vi "DCREG.vi"(10 "Simulazione":bool) -> ()   [LabVIEW 2019]
uses:
  Parametri DCREG letti.ctl
  <vilib>/Utility/file.llb/Read Delimited Spreadsheet (string).vi
  <vilib>/Modbus/master/Create Master Instance (Serial).vi
  Global FINE AVVIO.vi
  <vilib>/Modbus/master/Modbus Master.lvclass
  <vilib>/ptbypt/NI_PtbyPt.lvlib
panel:
  out "# elements in queue":i32
  out "P010 RPM max":dbl
  out "Connesso?":bool=TRUE
  out "Configurazioni dcreg":T1
  out "error out 5":errorcluster
  out "error out 4":errorcluster
  out "error out 3":errorcluster
  out "error out 2":errorcluster
  out "M0018 I CAMPO [A]":dbl
  out "M006 V ARMATURA [V]":dbl
  out "M004 I ARMATURA [A]":dbl
  out "P011 Vdc arm NOM":dbl
  in  "config":bool
  in  "Config DCreg":T1
  in  "IECC":dbl
  in  "SET IECC":bool
  in  "set rampa":bool
  in  "Rampa s":dbl
  in  "set Iarm":bool
  in  "Inom arm":dbl
  in  "set varm":bool
  in  "Vdc arm":dbl
  in  "disconnetti":bool
  in  "connetti":bool
  out "Iecc":dbl
  out "Iecc":dbl
  out "Imax mot":dbl
  out "Vdcreg":dbl
  in  "Leggi tutto?":bool
  out "P[KW]":dbl
  out "I[A]":dbl
  out "V[V]":dbl
  out "error out":errorcluster
  out "DCREG":T2
  in  "starting address":u16
  in  "holding register values":u16[](array[numeric])
  out "t":errorcluster
  out "N°reg_ValReg":i32[][](array[numeric])
  in  "mostra num registro":bool
  in  "SETUP PORTA SERIALE":T3={"Porta COM"="COM8", "Baud Rate"=38400, "Parity"=0, "Flow Control"=0, "Timeout"=10000, "Mode"=enum."RTU", "Slave Address"=2} {"Flow Control" items=["None", "XON/XOFF", "RTS/CTS", "XON/XOFF & RTS/CTS", "DTR/DSR", "XON/XOFF & DTR/DSR"]; "Parity" items=["None", "Odd", "Even", "Mark", "Space"]}
  out "STATO":string
  out "Numeric":i32
  in  "stop":bool
  in  "write register":bool
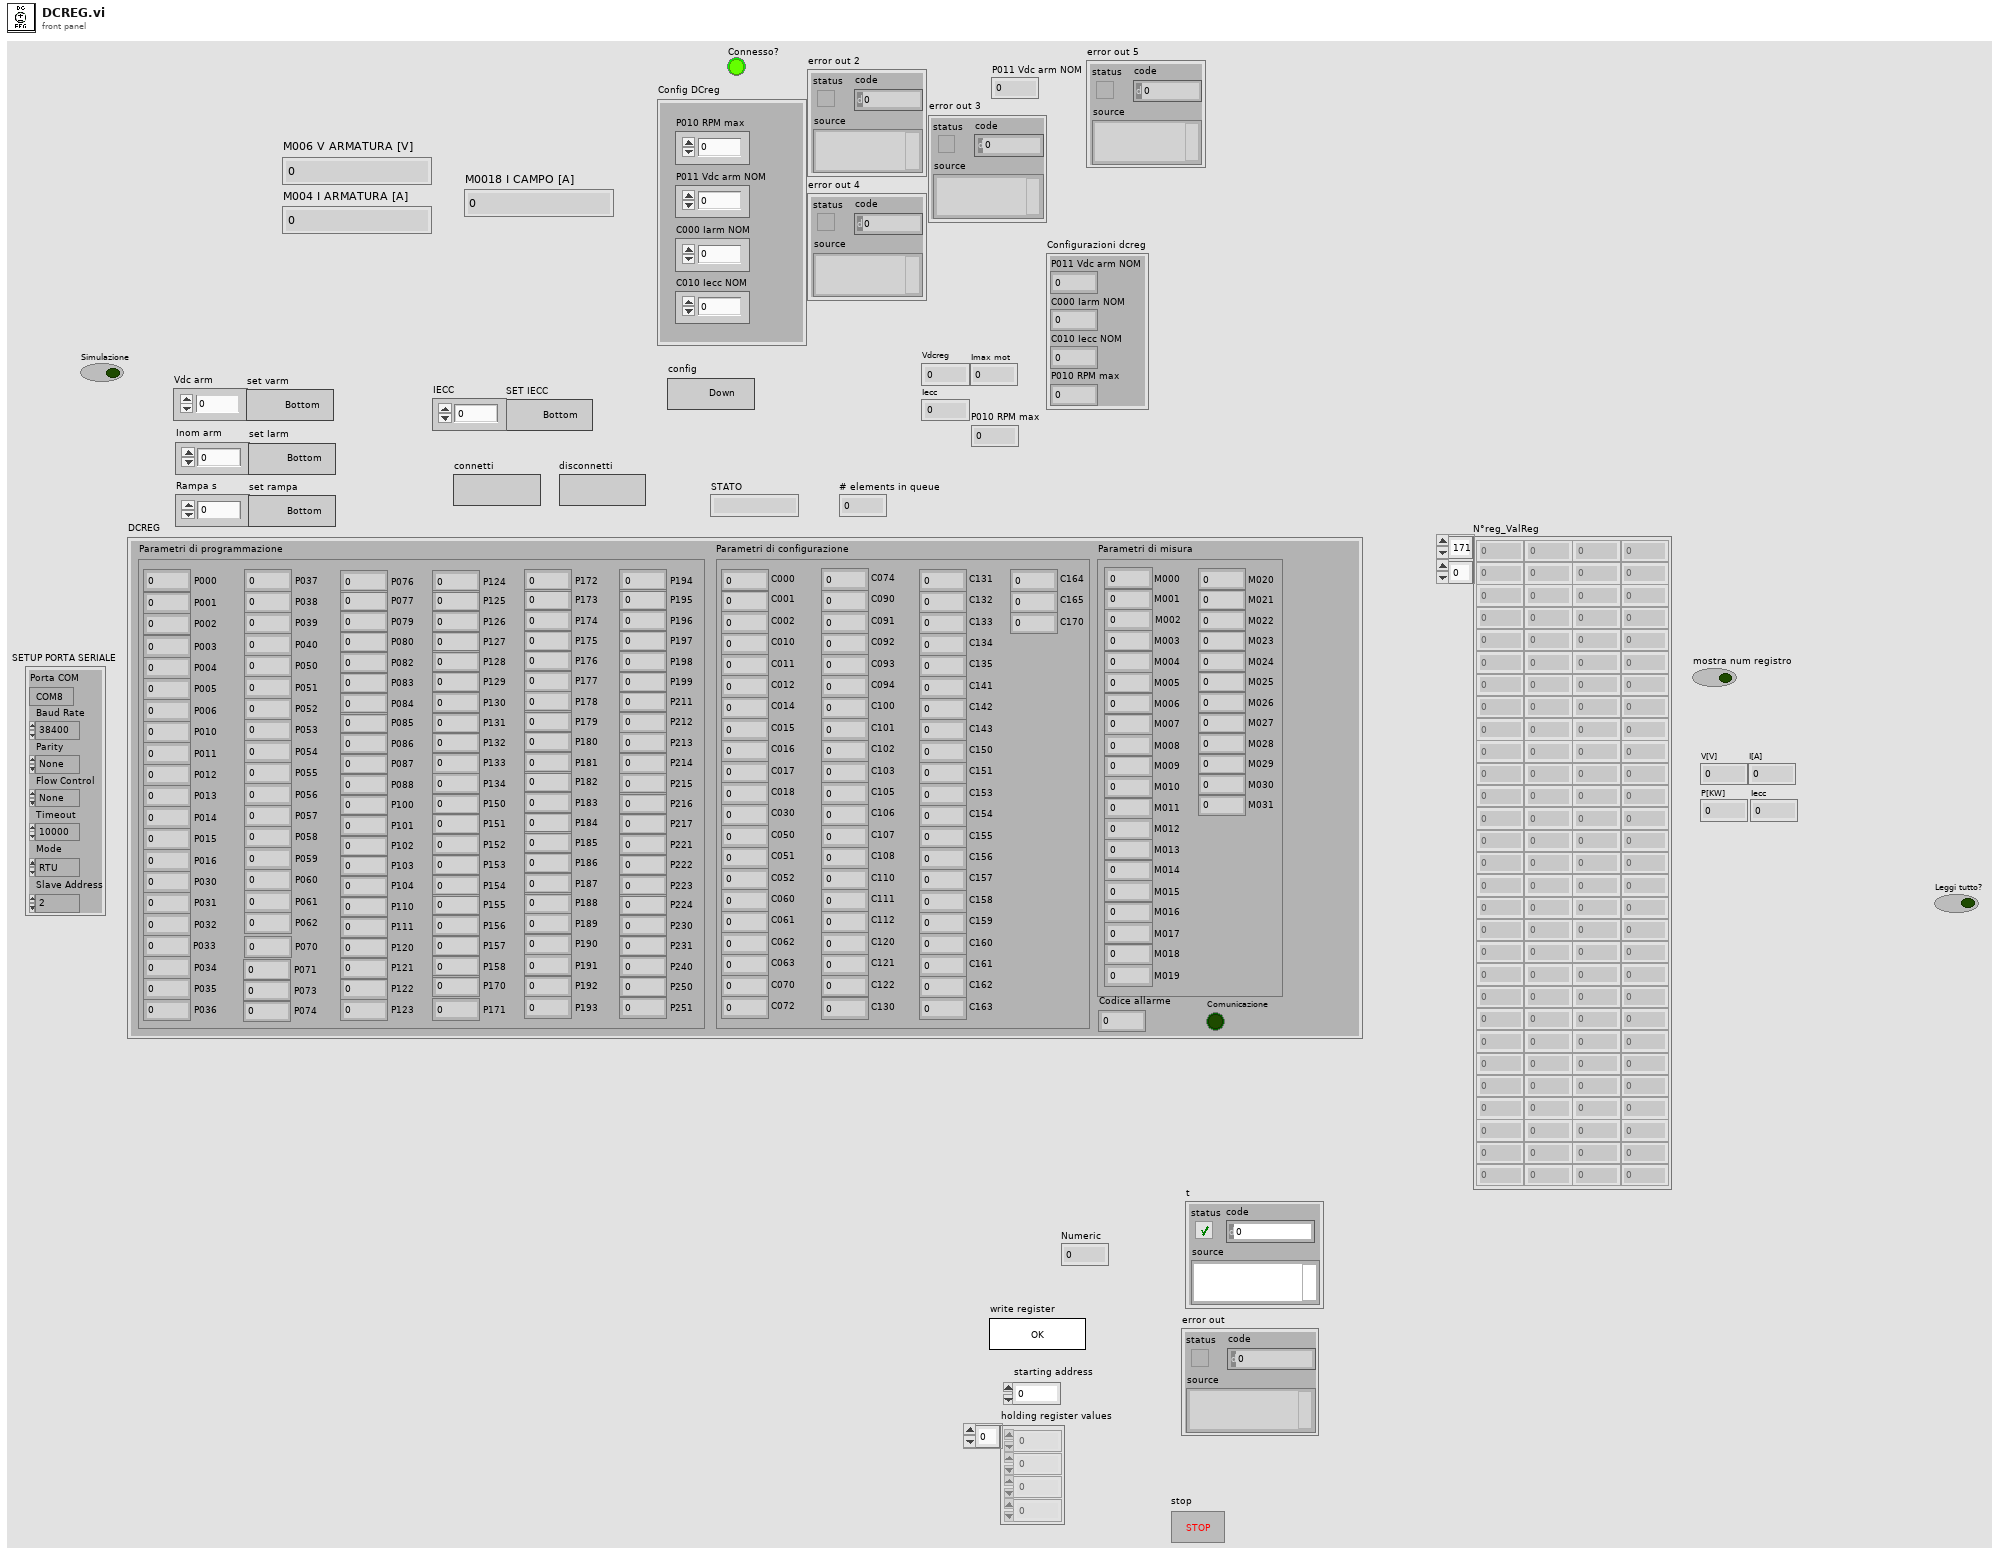
[diagram p1: front panel]
types:
  T1 = cluster{"P011 Vdc arm NOM":dbl, "C000 Iarm NOM":dbl, "C010 Iecc NOM":dbl, "P010 RPM max":dbl}
  T2 = typedef "Parametri DCREG letti.ctl" = cluster{"Parametri di misura":cluster{"M000":dbl, "M001":dbl, "M002":dbl, "M003":dbl, "M004":dbl, "M005":dbl, "M006":dbl, "M007":dbl, "M008":dbl, "M009":dbl, "M010":dbl, "M011":dbl, "M012":dbl, "M013":dbl, "M014":dbl, "M015":dbl, "M016":dbl, "M017":dbl, "M018":dbl, "M019":dbl, "M020":dbl, "M021":dbl, "M022":dbl, "M023":dbl, "M024":dbl, "M025":dbl, "M026":dbl, "M027":dbl, "M028":dbl, "M029":dbl, "M030":dbl, "M031":dbl}, "Parametri di programmazione":cluster{"P000":dbl, "P001":dbl, "P002":dbl, "P003":dbl, "P004":dbl, "P005":dbl, "P006":dbl, "P010":dbl, "P011":dbl, "P012":dbl, "P013":dbl, "P014":dbl, "P015":dbl, "P016":dbl, "P030":dbl, "P031":dbl, "P032":dbl, "P033":dbl, "P034":dbl, "P035":dbl, "P036":dbl, "P037":dbl, "P038":dbl, "P039":dbl, "P040":dbl, "P050":dbl, "P051":dbl, "P052":dbl, "P053":dbl, "P054":dbl, "P055":dbl, "P056":dbl, "P057":dbl, "P058":dbl, "P059":dbl, "P060":dbl, "P061":dbl, "P062":dbl, "P070":dbl, "P071":dbl, "P073":dbl, "P074":dbl, "P076":dbl, "P077":dbl, "P079":dbl, "P080":dbl, "P082":dbl, "P083":dbl, "P084":dbl, "P085":dbl, "P086":dbl, "P087":dbl, "P088":dbl, "P100":dbl, "P101":dbl, "P102":dbl, "P103":dbl, "P104":dbl, "P110":dbl, "P111":dbl, "P120":dbl, "P121":dbl, "P122":dbl, "P123":dbl, "P124":dbl, "P125":dbl, "P126":dbl, "P127":dbl, "P128":dbl, "P129":dbl, "P130":dbl, "P131":dbl, "P132":dbl, "P133":dbl, "P134":dbl, "P150":dbl, "P151":dbl, "P152":dbl, "P153":dbl, "P154":dbl, "P155":dbl, "P156":dbl, "P157":dbl, "P158":dbl, "P170":dbl, "P171":dbl, "P172":dbl, "P173":dbl, "P174":dbl, "P175":dbl, "P176":dbl, "P177":dbl, "P178":dbl, "P179":dbl, "P180":dbl, "P181":dbl, "P182":dbl, "P183":dbl, "P184":dbl, "P185":dbl, "P186":dbl, "P187":dbl, "P188":dbl, "P189":dbl, "P190":dbl, "P191":dbl, "P192":dbl, "P193":dbl, "P194":dbl, "P195":dbl, "P196":dbl, "P197":dbl, "P198":dbl, "P199":dbl, "P211":dbl, "P212":dbl, "P213":dbl, "P214":dbl, "P215":dbl, "P216":dbl, "P217":dbl, "P221":dbl, "P222":dbl, "P223":dbl, "P224":dbl, "P230":dbl, "P231":dbl, "P240":dbl, "P250":dbl, "P251":dbl}, "Parametri di configurazione":cluster{"C000":dbl, "C001":dbl, "C002":dbl, "C010":dbl, "C011":dbl, "C012":dbl, "C014":dbl, "C015":dbl, "C016":dbl, "C017":dbl, "C018":dbl, "C030":dbl, "C050":dbl, "C051":dbl, "C052":dbl, "C060":dbl, "C061":dbl, "C062":dbl, "C063":dbl, "C070":dbl, "C072":dbl, "C074":dbl, "C090":dbl, "C091":dbl, "C092":dbl, "C093":dbl, "C094":dbl, "C100":dbl, "C101":dbl, "C102":dbl, "C103":dbl, "C105":dbl, "C106":dbl, "C107":dbl, "C108":dbl, "C110":dbl, "C111":dbl, "C112":dbl, "C120":dbl, "C121":dbl, "C122":dbl, "C130":dbl, "C131":dbl, "C132":dbl, "C133":dbl, "C134":dbl, "C135":dbl, "C141":dbl, "C142":dbl, "C143":dbl, "C150":dbl, "C151":dbl, "C153":dbl, "C154":dbl, "C155":dbl, "C156":dbl, "C157":dbl, "C158":dbl, "C159":dbl, "C160":dbl, "C161":dbl, "C162":dbl, "C163":dbl, "C164":dbl, "C165":dbl, "C170":dbl}, "Codice allarme":dbl, "Comunicazione":bool}
  T3 = cluster{"Porta COM":string, "Baud Rate":u32, "Parity":u16, "Flow Control":u16, "Timeout":u32, "Mode":enum16{"RTU", "ASCII"}, "Slave Address":u8}
  T4 = cluster{"Array of elements":cluster{"String":string, "variant":variant}[], "Single element":cluster{"String":string, "variant":variant}, "enque at\nopposite end (F)":bool, "no replications (F)":bool}
  T5 = cluster{"P000":dbl, "P001":dbl, "P002":dbl, "P003":dbl, "P004":dbl, "P005":dbl, "P006":dbl, "P010":dbl, "P011":dbl, "P012":dbl, "P013":dbl, "P014":dbl, "P015":dbl, "P016":dbl, "P030":dbl, "P031":dbl, "P032":dbl, "P033":dbl, "P034":dbl, "P035":dbl, "P036":dbl, "P037":dbl, "P038":dbl, "P039":dbl, "P040":dbl, "P050":dbl, "P051":dbl, "P052":dbl, "P053":dbl, "P054":dbl, "P055":dbl, "P056":dbl, "P057":dbl, "P058":dbl, "P059":dbl, "P060":dbl, "P061":dbl, "P062":dbl, "P070":dbl, "P071":dbl, "P073":dbl, "P074":dbl, "P076":dbl, "P077":dbl, "P079":dbl, "P080":dbl, "P082":dbl, "P083":dbl, "P084":dbl, "P085":dbl, "P086":dbl, "P087":dbl, "P088":dbl, "P100":dbl, "P101":dbl, "P102":dbl, "P103":dbl, "P104":dbl, "P110":dbl, "P111":dbl, "P120":dbl, "P121":dbl, "P122":dbl, "P123":dbl, "P124":dbl, "P125":dbl, "P126":dbl, "P127":dbl, "P128":dbl, "P129":dbl, "P130":dbl, "P131":dbl, "P132":dbl, "P133":dbl, "P134":dbl, "P150":dbl, "P151":dbl, "P152":dbl, "P153":dbl, "P154":dbl, "P155":dbl, "P156":dbl, "P157":dbl, "P158":dbl, "P170":dbl, "P171":dbl, "P172":dbl, "P173":dbl, "P174":dbl, "P175":dbl, "P176":dbl, "P177":dbl, "P178":dbl, "P179":dbl, "P180":dbl, "P181":dbl, "P182":dbl, "P183":dbl, "P184":dbl, "P185":dbl, "P186":dbl, "P187":dbl, "P188":dbl, "P189":dbl, "P190":dbl, "P191":dbl, "P192":dbl, "P193":dbl, "P194":dbl, "P195":dbl, "P196":dbl, "P197":dbl, "P198":dbl, "P199":dbl, "P211":dbl, "P212":dbl, "P213":dbl, "P214":dbl, "P215":dbl, "P216":dbl, "P217":dbl, "P221":dbl, "P222":dbl, "P223":dbl, "P224":dbl, "P230":dbl, "P231":dbl, "P240":dbl, "P250":dbl, "P251":dbl}
  T6 = cluster{"C000":dbl, "C001":dbl, "C002":dbl, "C010":dbl, "C011":dbl, "C012":dbl, "C014":dbl, "C015":dbl, "C016":dbl, "C017":dbl, "C018":dbl, "C030":dbl, "C050":dbl, "C051":dbl, "C052":dbl, "C060":dbl, "C061":dbl, "C062":dbl, "C063":dbl, "C070":dbl, "C072":dbl, "C074":dbl, "C090":dbl, "C091":dbl, "C092":dbl, "C093":dbl, "C094":dbl, "C100":dbl, "C101":dbl, "C102":dbl, "C103":dbl, "C105":dbl, "C106":dbl, "C107":dbl, "C108":dbl, "C110":dbl, "C111":dbl, "C112":dbl, "C120":dbl, "C121":dbl, "C122":dbl, "C130":dbl, "C131":dbl, "C132":dbl, "C133":dbl, "C134":dbl, "C135":dbl, "C141":dbl, "C142":dbl, "C143":dbl, "C150":dbl, "C151":dbl, "C153":dbl, "C154":dbl, "C155":dbl, "C156":dbl, "C157":dbl, "C158":dbl, "C159":dbl, "C160":dbl, "C161":dbl, "C162":dbl, "C163":dbl, "C164":dbl, "C165":dbl, "C170":dbl}
  T7 = cluster{"M000":dbl, "M001":dbl, "M002":dbl, "M003":dbl, "M004":dbl, "M005":dbl, "M006":dbl, "M007":dbl, "M008":dbl, "M009":dbl, "M010":dbl, "M011":dbl, "M012":dbl, "M013":dbl, "M014":dbl, "M015":dbl, "M016":dbl, "M017":dbl, "M018":dbl, "M019":dbl, "M020":dbl, "M021":dbl, "M022":dbl, "M023":dbl, "M024":dbl, "M025":dbl, "M026":dbl, "M027":dbl, "M028":dbl, "M029":dbl, "M030":dbl, "M031":dbl}
  T8 = cluster{"C011":dbl, "C012":dbl, "C016":dbl, "Conferma":bool}
  T9 = cluster{"[0]":i32, "[1]":i32, "[2]":i32, "[3]":i32, "[4]":i32, "[5]":i32, "[6]":i32, "[7]":i32, "[8]":i32, "[9]":i32, "[10]":i32, "[11]":i32, "[12]":i32, "[13]":i32, "[14]":i32, "[15]":i32, "[16]":i32, "[17]":i32, "[18]":i32, "[19]":i32, "[20]":i32, "[21]":i32, "[22]":i32, "[23]":i32, "[24]":i32, "[25]":i32, "[26]":i32, "[27]":i32, "[28]":i32, "[29]":i32, "[30]":i32, "[31]":i32}
  T10 = cluster{"[0]":i32, "[1]":i32, "[2]":i32, "[3]":i32, "[4]":i32, "[5]":i32, "[6]":i32, "[7]":i32, "[8]":i32, "[9]":i32, "[10]":i32, "[11]":i32, "[12]":i32, "[13]":i32, "[14]":i32, "[15]":i32, "[16]":i32, "[17]":i32, "[18]":i32, "[19]":i32, "[20]":i32, "[21]":i32, "[22]":i32, "[23]":i32, "[24]":i32, "[25]":i32, "[26]":i32, "[27]":i32, "[28]":i32, "[29]":i32, "[30]":i32, "[31]":i32, "[32]":i32, "[33]":i32, "[34]":i32, "[35]":i32, "[36]":i32, "[37]":i32, "[38]":i32, "[39]":i32, "[40]":i32, "[41]":i32, "[42]":i32, "[43]":i32, "[44]":i32, "[45]":i32, "[46]":i32, "[47]":i32, "[48]":i32, "[49]":i32, "[50]":i32, "[51]":i32, "[52]":i32, "[53]":i32, "[54]":i32, "[55]":i32, "[56]":i32, "[57]":i32, "[58]":i32, "[59]":i32, "[60]":i32, "[61]":i32, "[62]":i32, "[63]":i32, "[64]":i32, "[65]":i32, "[66]":i32, "[67]":i32, "[68]":i32, "[69]":i32, "[70]":i32, "[71]":i32, "[72]":i32, "[73]":i32, "[74]":i32, "[75]":i32, "[76]":i32, "[77]":i32, "[78]":i32, "[79]":i32, "[80]":i32, "[81]":i32, "[82]":i32, "[83]":i32, "[84]":i32, "[85]":i32, "[86]":i32, "[87]":i32, "[88]":i32, "[89]":i32, "[90]":i32, "[91]":i32, "[92]":i32, "[93]":i32, "[94]":i32, "[95]":i32, "[96]":i32, "[97]":i32, "[98]":i32, "[99]":i32, "[100]":i32, "[101]":i32, "[102]":i32, "[103]":i32, "[104]":i32, "[105]":i32, "[106]":i32, "[107]":i32, "[108]":i32, "[109]":i32, "[110]":i32, "[111]":i32, "[112]":i32, "[113]":i32, "[114]":i32, "[115]":i32, "[116]":i32, "[117]":i32, "[118]":i32, "[119]":i32, "[120]":i32, "[121]":i32, "[122]":i32, "[123]":i32, "[124]":i32, "[125]":i32, "[126]":i32, "[127]":i32, "[128]":i32, "[129]":i32}
  T11 = cluster{"[0]":i32, "[1]":i32, "[2]":i32, "[3]":i32, "[4]":i32, "[5]":i32, "[6]":i32, "[7]":i32, "[8]":i32, "[9]":i32, "[10]":i32, "[11]":i32, "[12]":i32, "[13]":i32, "[14]":i32, "[15]":i32, "[16]":i32, "[17]":i32, "[18]":i32, "[19]":i32, "[20]":i32, "[21]":i32, "[22]":i32, "[23]":i32, "[24]":i32, "[25]":i32, "[26]":i32, "[27]":i32, "[28]":i32, "[29]":i32, "[30]":i32, "[31]":i32, "[32]":i32, "[33]":i32, "[34]":i32, "[35]":i32, "[36]":i32, "[37]":i32, "[38]":i32, "[39]":i32, "[40]":i32, "[41]":i32, "[42]":i32, "[43]":i32, "[44]":i32, "[45]":i32, "[46]":i32, "[47]":i32, "[48]":i32, "[49]":i32, "[50]":i32, "[51]":i32, "[52]":i32, "[53]":i32, "[54]":i32, "[55]":i32, "[56]":i32, "[57]":i32, "[58]":i32, "[59]":i32, "[60]":i32, "[61]":i32, "[62]":i32, "[63]":i32, "[64]":i32, "[65]":i32}
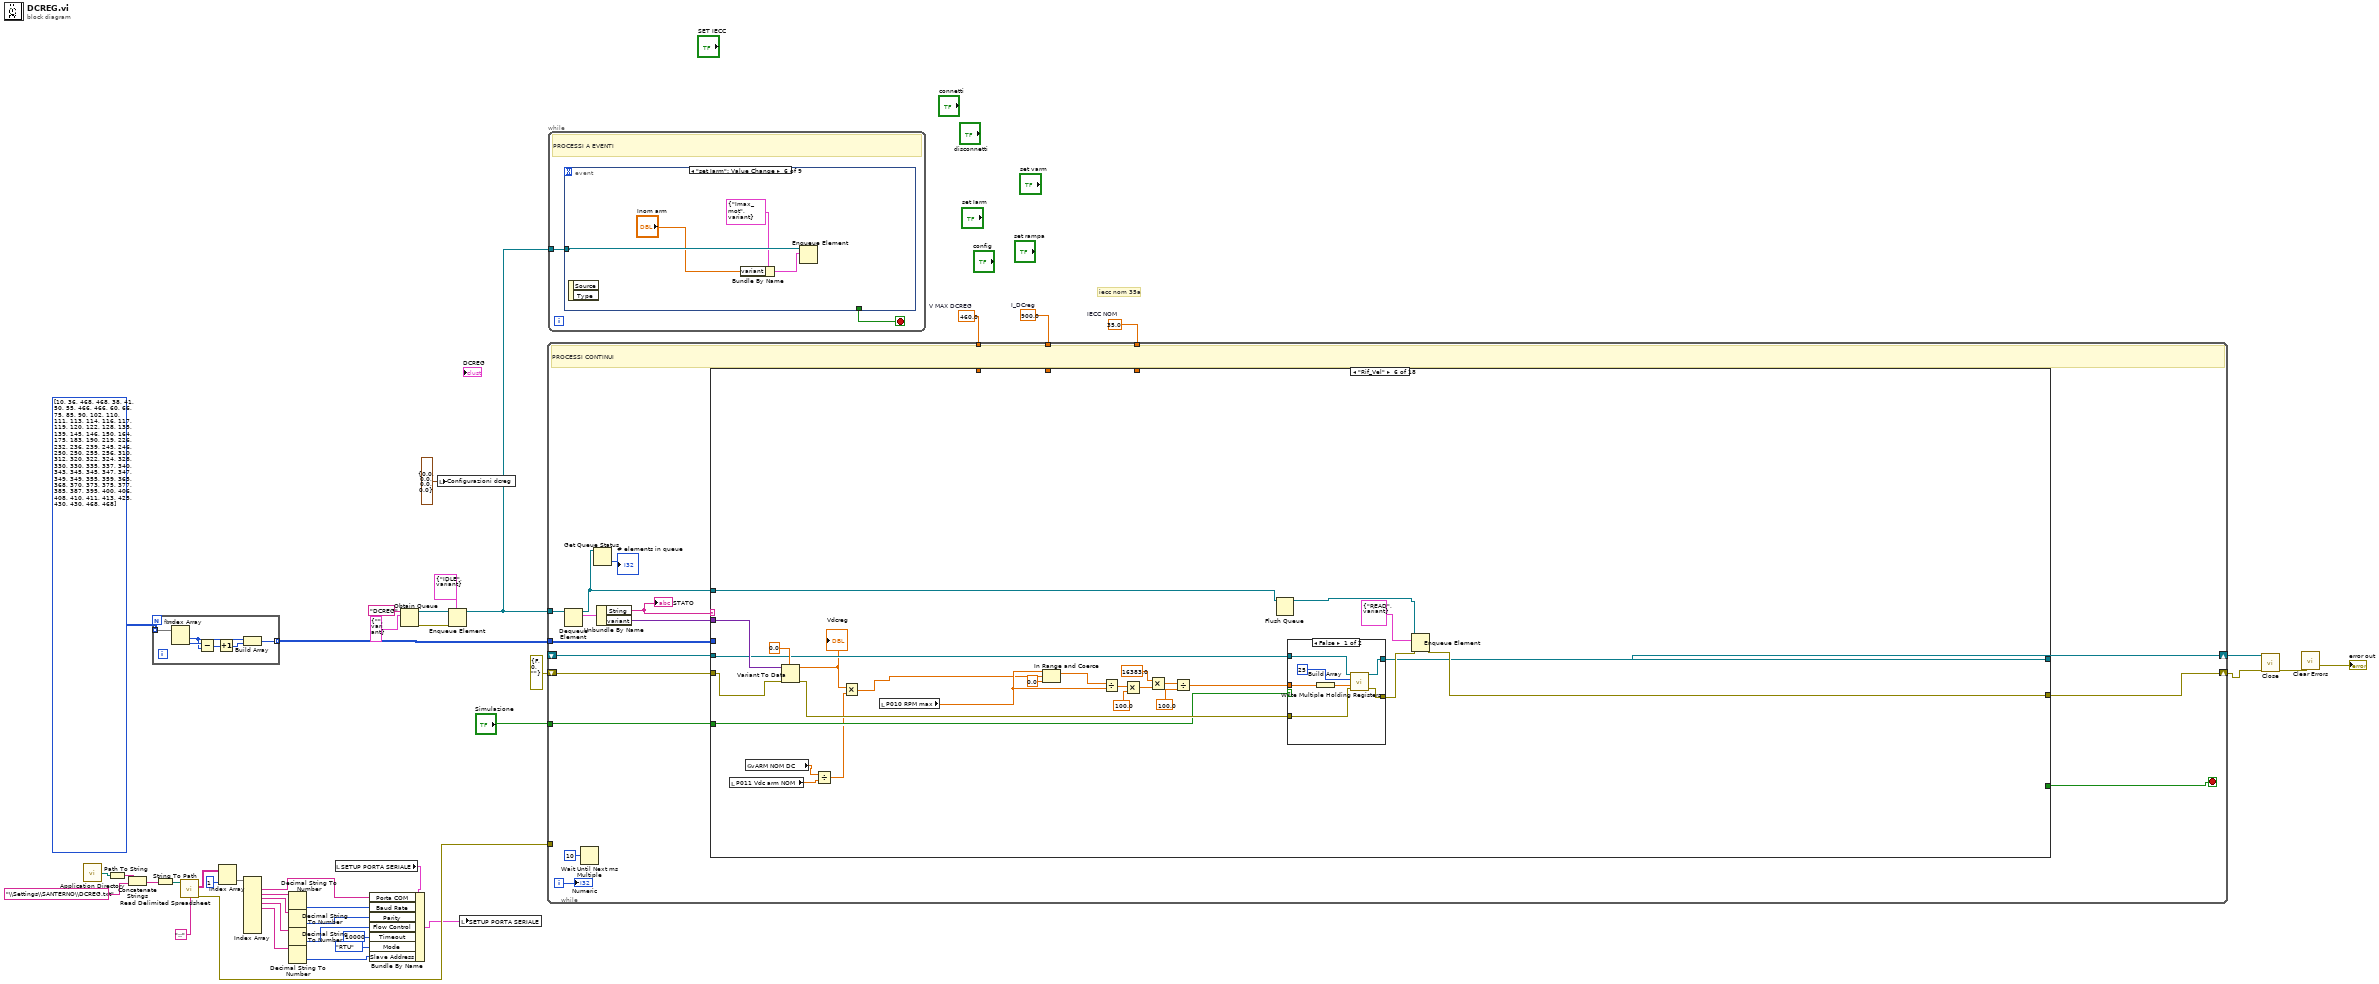
[diagram p0: block diagram]
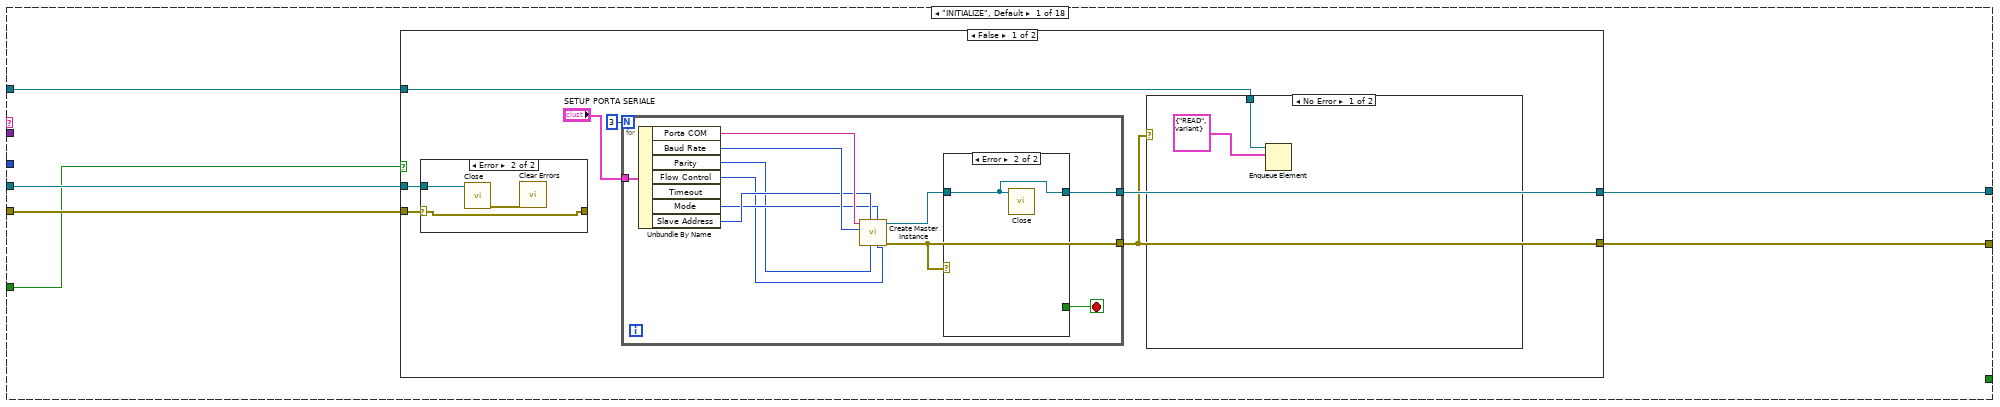
[diagram p2: hidden frame]
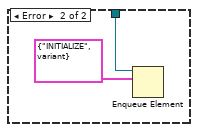
[diagram p3: hidden frame]
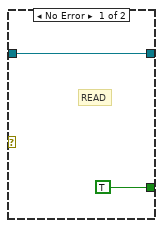
[diagram p5: hidden frame]
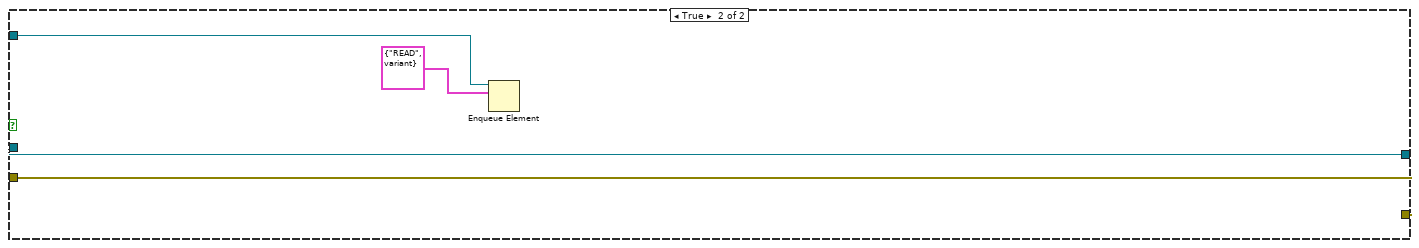
[diagram p6: hidden frame]
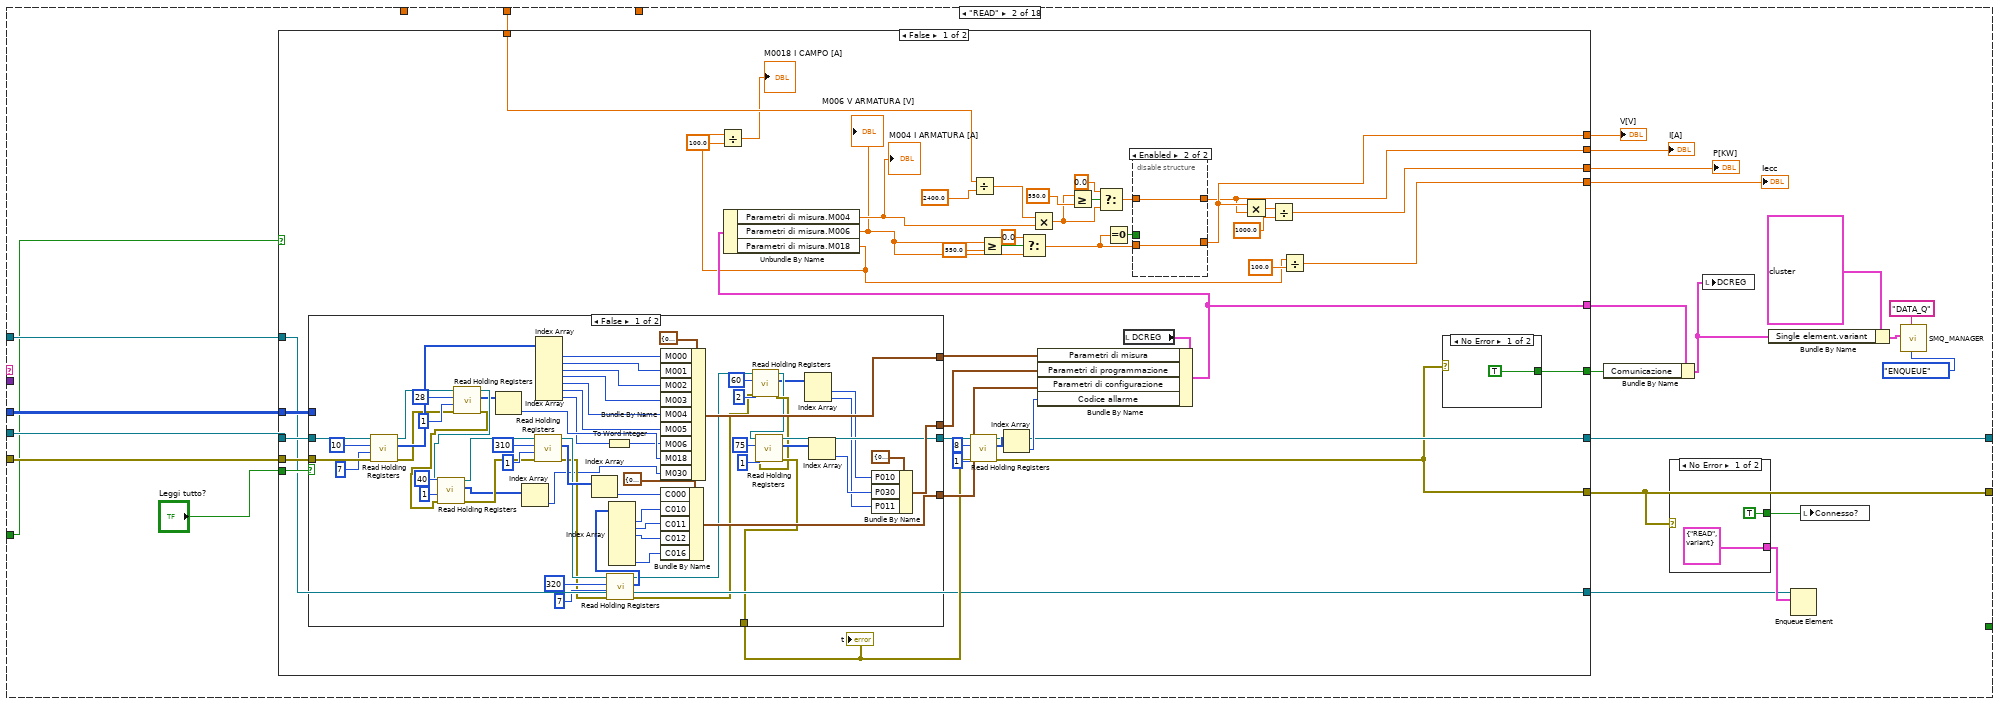
[diagram p7: hidden frame]
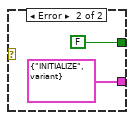
[diagram p8: hidden frame]
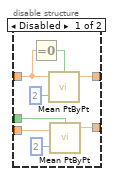
[diagram p10: hidden frame]
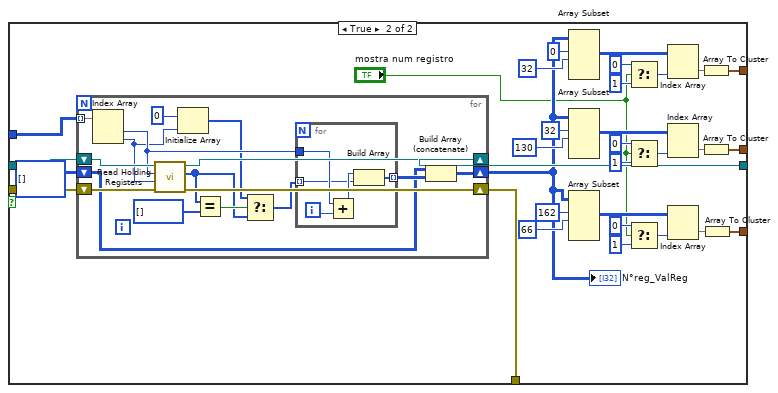
[diagram p11: hidden frame]
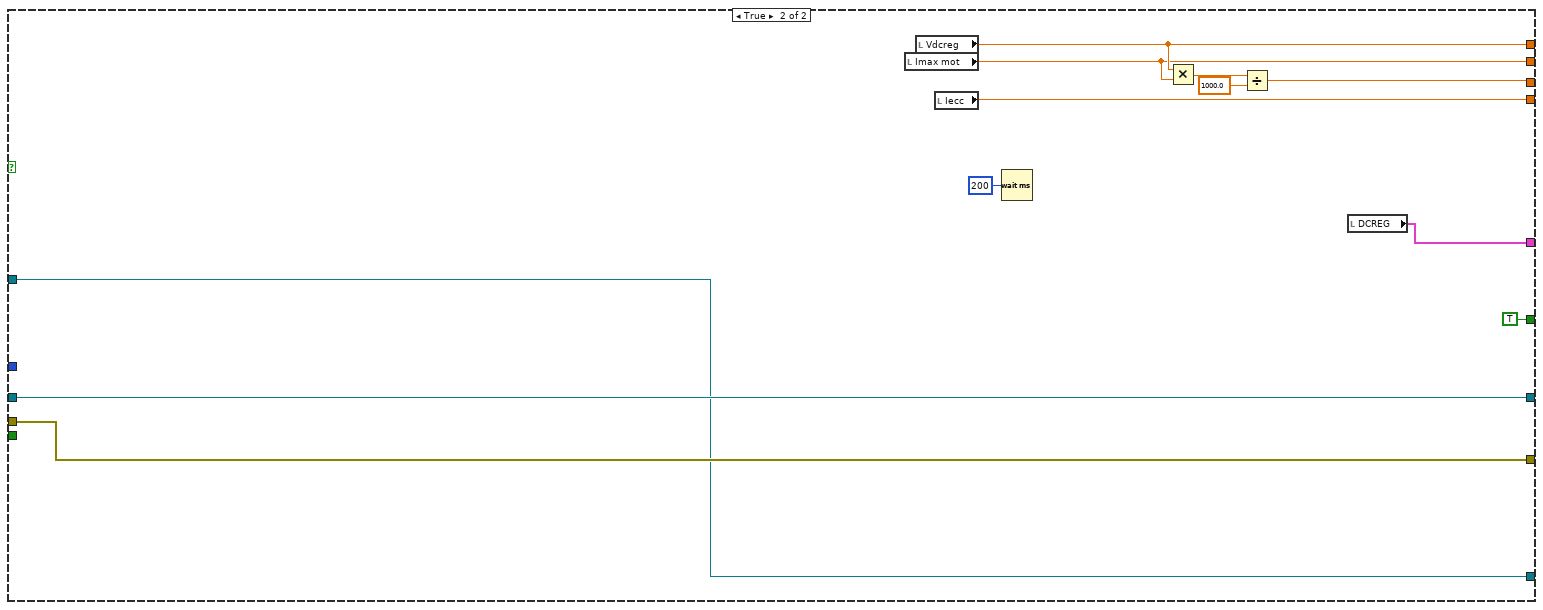
[diagram p12: hidden frame]
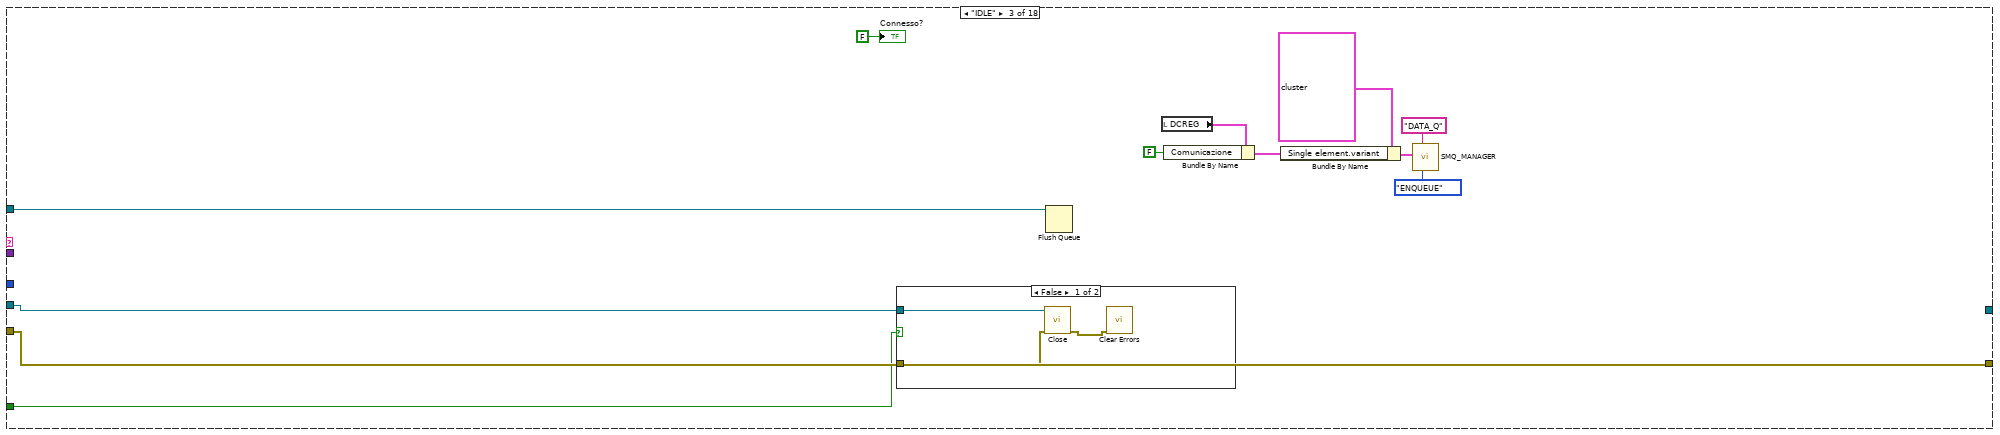
[diagram p13: hidden frame]
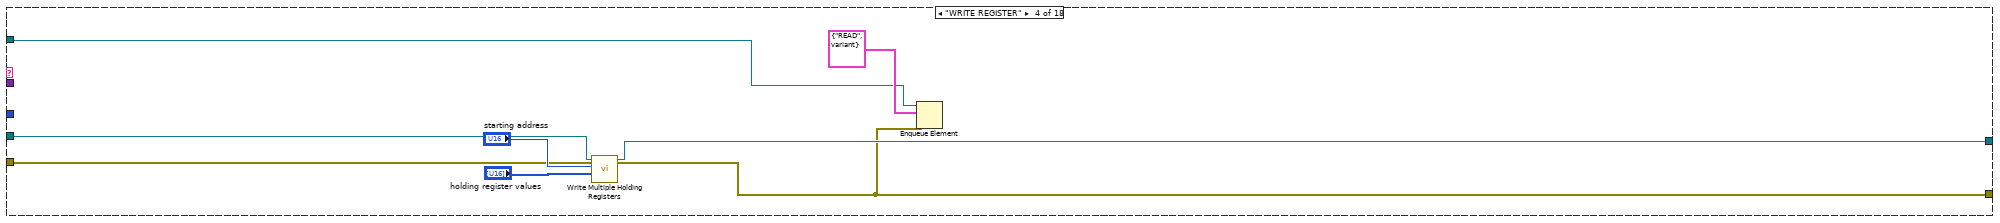
[diagram p15: hidden frame]
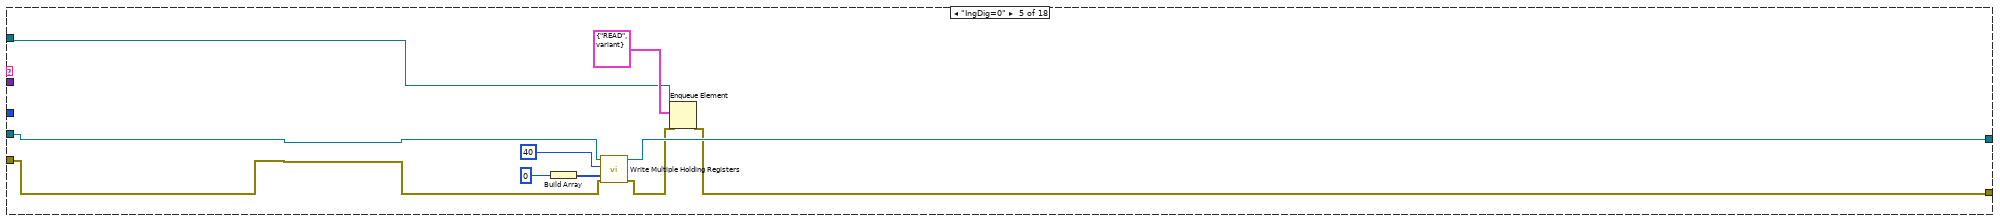
[diagram p16: hidden frame]
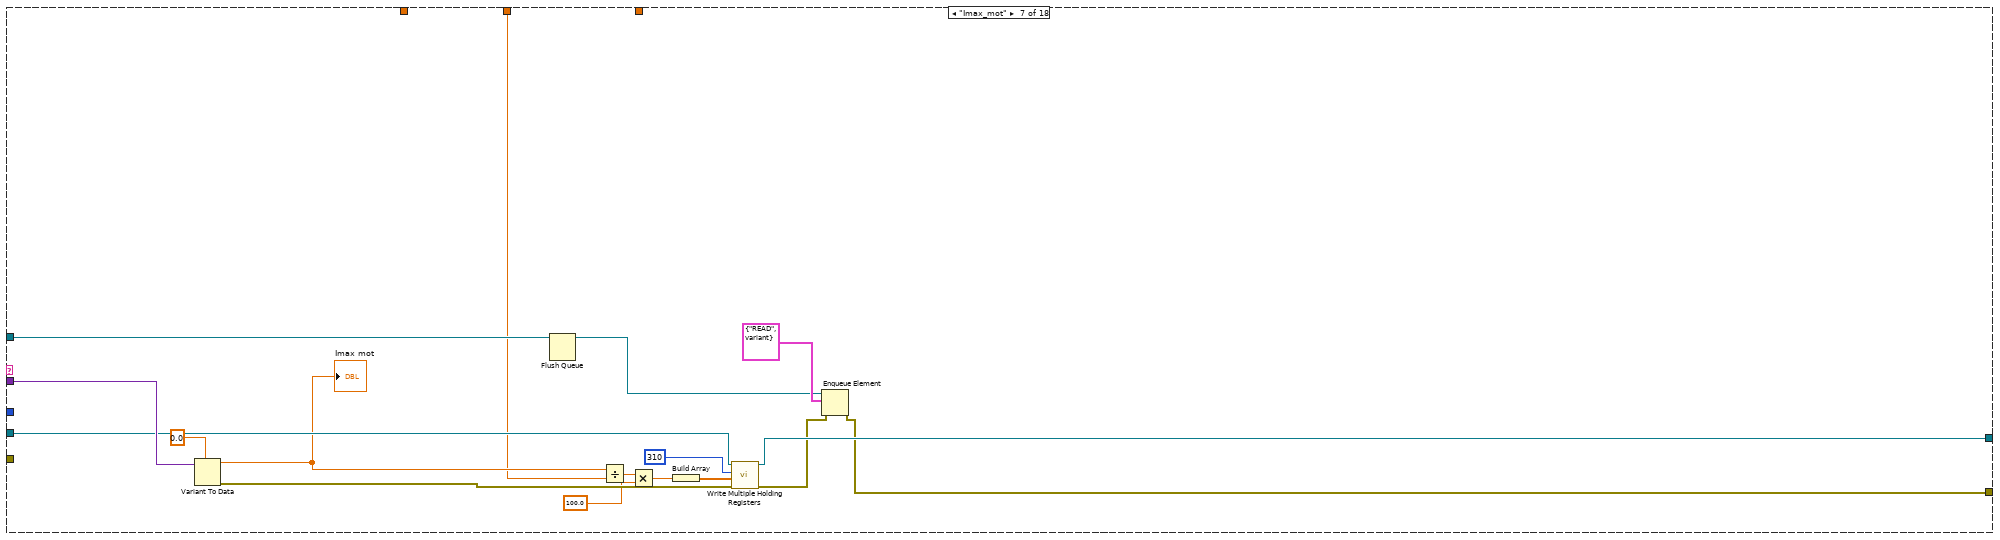
[diagram p18: hidden frame]
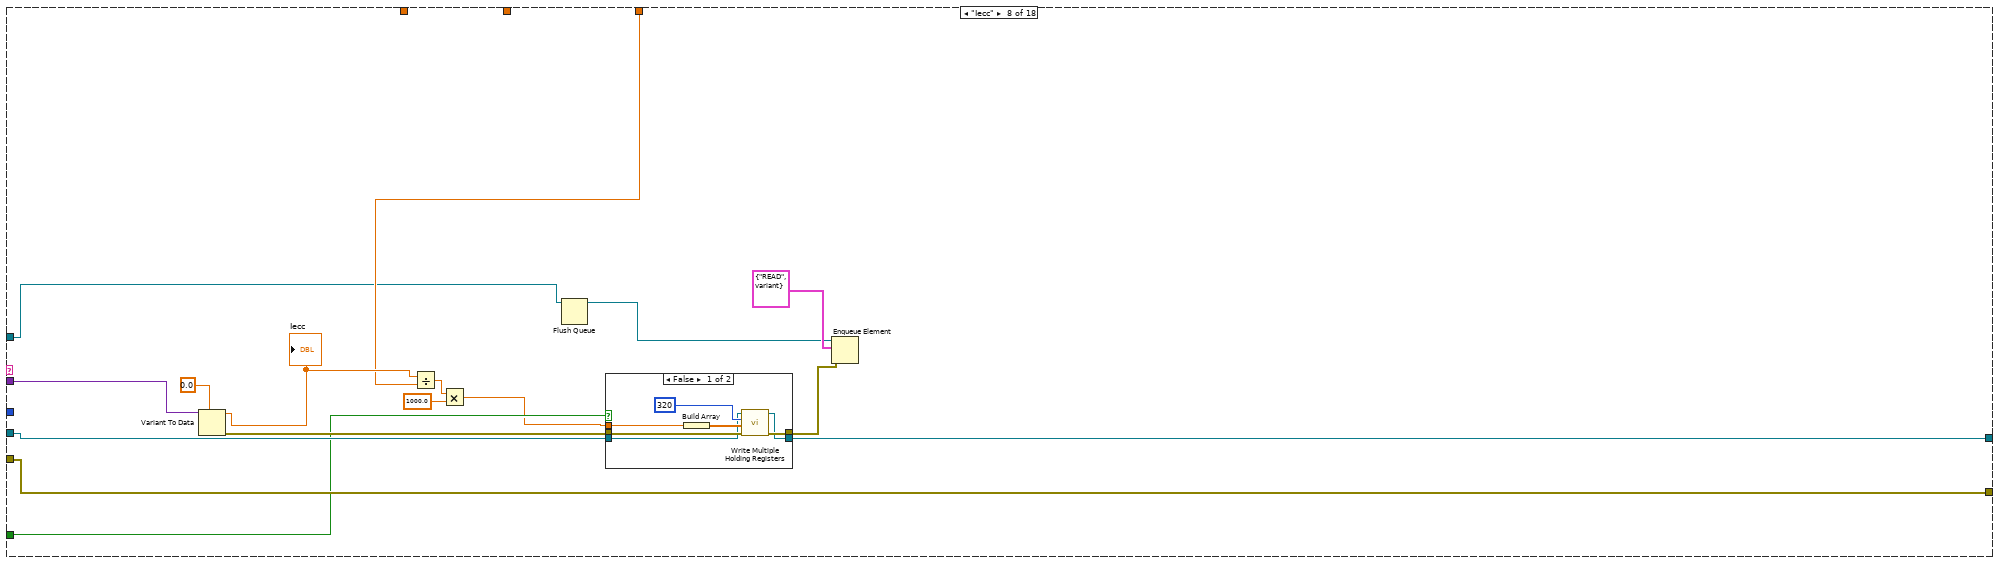
[diagram p19: hidden frame]
diagram:
  w25 = 35.0  # IECC NOM
  w29 = 900.0  # I_DCreg
  w30 = 460.0  # V MAX DCREG
  # "iecc nom 35a"
  n1 = call <vilib>:"Application Directory.vi"() -> ("Application Directory"=w12:path)
  n2 = Path To String(path=w12) -> (string=w13:string)
  n3 = Concatenate Strings(w13, "\\Settings\\SANTERNO\\DCREG.txt" ("string")) -> (w15:string)
  n4 = for {
    tunnel: i32[][] [[10, 36], [468, 468], [38, 41], [50, 55], [466, 466], [60, 66], [75, 85], [90, 102], [110, 111], [113, 114], [116, 117], [119, 120], [122, 128], [135, 139], [145, 146], [150, 164], [175, 183], [190, 219], [226, 232], [236, 239], [245, 246], [250, 250], [255, 256], [310, 312], [320, 322], [324, 328], [330, 330], [335, 337], [340, 343], [345, 345], [347, 347], [349, 349], [355, 359], [365, 368], [370, 373], [375, 377], [385, 387], [395, 400], [406, 408], [410, 411], [413, 425], [430, 430], [468, 468]] -> [w47] mode=indexing
    tunnel: [w42] -> w39 mode=indexing
    n5 = Index Array(array=w47) -> (element #1=w43:i32, element #2=w46:i32)  [unwired: 2 in]
    n6 = Subtract(x=w46, y=w43) -> (x-y=w45:i32)
    n7 = Increment(x=w45) -> (x+1=w44:i32)
    n8 = Build Array(w43, w44) -> (w42:i32[])
  }
  n9 = String To Path(string=w15) -> (path=w16:path)
  n10 = call-poly <vilib>:"Read Delimited Spreadsheet.vi"("file path (dialog if empty)"=w16, "delimiter (\\t)"="::" ("delimiter (\\t)")) -> ("all rows"=w17:string[][], "error out"=w3:errorcluster)  [unwired: 8 in, 4 out]
  n11 = Index Array(array=w17, index (col)=1 ("disabled index (col)")) -> (element=w19:string[])  [unwired: 1 in]
  n12 = Index Array(array=w19) -> (element #1=w10:string, element #2=w20:string, element #3=w21:string, element #4=w22:string, element #5=w23:string)  [unwired: 10 in, 5 out]
  n13 = Decimal String To Number(string=w20) -> (number=w9:i32)  [unwired: 2 in, 1 out]
  n14 = Decimal String To Number(string=w21) -> (number=w8:i32)  [unwired: 2 in, 1 out]
  n15 = Decimal String To Number(string=w22) -> (number=w7:i32)  [unwired: 2 in, 1 out]
  n16 = Decimal String To Number(string=w23) -> (number=w5:i32)  [unwired: 2 in, 1 out]
  n17 = local read "SETUP PORTA SERIALE"() -> (w1:T3)
  n18 = Bundle By Name(cluster=w1, "Porta COM"=w10, "Baud Rate"=w9, "Parity"=w8, "Flow Control"=w7, "Timeout"=u32 10000, "Mode"=enum16{"RTU", "ASCII"}."RTU", "Slave Address"=w5) -> (w2:T3)
  n19 = Obtain Queue(name (unnamed)="DCREG", element data type=cluster{"String":string, "variant":variant} {"String"="", "variant"=variant} ("element")) -> (queue out=w31:refnum<queue>, error out=w33:errorcluster)  [unwired: 3 in, 1 out]
  n20 = local write "Configurazioni dcreg"(T1 {"P011 Vdc arm NOM"=0.0, "C000 Iarm NOM"=0.0, "C010 Iecc NOM"=0.0, "P010 RPM max"=0.0} ("Configurazioni dcreg")) -> ()
  n21 = Enqueue Element(queue=w31, element=cluster{"String":string, "variant":variant} {"String"="IDLE", "variant"=variant}, error in (no error)=w33) -> (queue out=w41:refnum<queue>)  [unwired: 1 in, 2 out]
  n22 = local write "SETUP PORTA SERIALE"(w2) -> ()
  n23 = while {
    shift-right: [w57] -> w37
    shift-left: errorcluster {"status"=FALSE, "code"=0, "source"=""} ("error out") -> [w65]
    tunnel: w41 -> [w55]
    shift-right: [w63] -> w38
    shift-left: _ -> [w62]
    tunnel: w39 -> [w61]
    tunnel: w30 -> [w59]
    tunnel: w29 -> [w58]
    tunnel: "Simulazione" -> [w51]
    tunnel: w25 -> [w50]
    tunnel: w3 -> [_]
    i -> [w64]
    stop <- w56 stop-if-true
    # "PROCESSI CONTINUI"
    n24 = Dequeue Element(queue=w55) -> (queue out=w49:refnum<queue>, element=w54:cluster{"String":string, "variant":variant})  [unwired: 2 in, 2 out]
    n25 = Wait Until Next ms Multiple(millisecond multiple=u32 10 ("milliseconds to wait")) -> ()  [unwired: 1 out]
    n26 = Get Queue Status(queue=w49) -> (# elements in queue=→"# elements in queue":i32)  [unwired: 2 in, 7 out]
    n27 = Unbundle By Name(w54) -> ("String"=w53:string, "variant"=w52:variant)
    "STATO" <- w53
    n28 = case shown="\"Rif_Vel\"" w53 {
      tunnel: [_ _ _ _ _ _ _ _ _ _ _ _ _ _ _ _ _ TRUE] -> w56
      tunnel: w65 -> [w69 w125 w322 w329 w335 w368 _ w413 _ w474 w490 w500 w511 w532 w538 w571 w617 w625]
      tunnel: [w67 w117 w322 w329 w337 w369 w388 w413 w426 w474 w478 w496 w506 w529 w541 w574 w614 w625] -> w57
      tunnel: w52 -> [_ _ _ _ _ w366 w393 w408 _ w471 w495 _ _ _ _ _ w622 _]
      tunnel: w49 -> [w68 w127 w324 w328 w343 w351 w387 w399 _ w468 _ w498 w508 w530 w542 w573 _ _]
      tunnel: [w71 w126 _ w331 w342 w363 w391 w406 w445 w473 w480 w499 w509 w525 w540 w575 w612 w624] -> w63
      tunnel: w62 -> [w70 w123 w323 w334 w336 w364 w392 w407 w457 w473 w491 w501 w510 w531 w539 w572 w619 w624]
      tunnel: w61 -> [_ w124 _ _ _ _ _ _ _ _ _ _ _ _ _ _ _ _]
      tunnel: w59 -> [_ _ _ _ _ _ _ _ _ _ _ _ _ _ _ _ _ _]
      tunnel: w58 -> [_ w121 _ _ _ _ w382 _ _ _ _ _ _ _ _ _ _ _]
      tunnel: w51 -> [w66 w120 w321 _ _ w355 _ w405 _ _ _ _ _ _ _ _ _ _]
      tunnel: w50 -> [_ _ _ _ _ _ _ w403 _ _ _ _ _ _ _ _ _ _]
      frame "INITIALIZE", Default {
        n29 = case shown="False" w66 {
          tunnel: [w76 w104] -> w71
          tunnel: w70 -> [w75 w104]
          tunnel: w69 -> [w74 w103]
          tunnel: w68 -> [w73 w101]
          tunnel: [w72 w103] -> w67
          frame False {
            n30 = case shown="Error" w74 {
              selector: w74 -> [w83 w85]
              tunnel: w75 -> [_ w86]
              tunnel: [w83 w85] -> _
              frame No Error {
              }
              frame Error {
                n31 = call-dynamic "Close.vi"("Modbus master in"=w86) -> ("error out"=w84:errorcluster)  [unwired: 10 in]
                n32 = call <vilib>:"Clear Errors.vi"("error in (no error)"=w84) -> ()  [unwired: 5 in, 2 out]
              }
            }
            n33 = for {
              N: 3 -> [_]
              tunnel: "SETUP PORTA SERIALE" -> [w97]
              tunnel: [w90] -> w72
              tunnel: [w88] -> w76
              stop <- w87 stop-if-true
              n34 = Unbundle By Name(w97) -> ("Porta COM"=w96:string, "Baud Rate"=w95:u32, "Parity"=w92:u16, "Flow Control"=w91:u16, "Mode"=w93:enum16{"RTU", "ASCII"}, "Slave Address"=w94:u8)  [unwired: 1 out]
              n35 = call-poly <vilib>:"Create Master Instance.vi"("flow control (None)"=w91, "serial type"=w93, "parity (Even)"=w92, "unit ID"=w94, "baud rate (9600)"=w95, "VISA resource name"=w96) -> ("error out"=w90:errorcluster, "serial master instance"=w89:refnum<class "Modbus Master.lvclass">)  [unwired: 4 in]
              n36 = case shown="Error" w90 {
                tunnel: w89 -> [w99 w100]
                tunnel: [w99 w100] -> w88
                tunnel: [TRUE _] -> w87
                frame No Error {
                  # "READ"
                }
                frame Error {
                  n37 = call-dynamic "Close.vi"("Modbus master in"=w100) -> ()  [unwired: 10 in, 1 out]
                }
              }
            }
            n38 = case shown="No Error" w72 {
              tunnel: w73 -> [w79 w81]
              frame No Error {
                n39 = Enqueue Element(queue=w79, element=cluster{"String":string, "variant":variant} {"String"="READ", "variant"=variant}) -> ()  [unwired: 2 in, 3 out]
              }
              frame Error {
                n40 = Enqueue Element(queue=w81, element=cluster{"String":string, "variant":variant} {"String"="INITIALIZE", "variant"=variant}) -> ()  [unwired: 2 in, 3 out]
              }
            }
          }
          frame True {
            n41 = Enqueue Element(queue=w101, element=cluster{"String":string, "variant":variant} {"String"="READ", "variant"=variant}) -> ()  [unwired: 2 in, 3 out]
          }
        }
      }
      frame "READ" {
        n42 = case shown="False" w120 {
          tunnel: w127 -> [w146 w310]
          tunnel: w124 -> [w175 _]
          tunnel: [w149 w312] -> w126
          tunnel: w123 -> [w174 w312]
          tunnel: w125 -> [w173 w311]
          tunnel: [w139 w311] -> w117
          tunnel: "Leggi tutto?" -> [w158 _]
          tunnel: w121 -> [w147 _]
          tunnel: [w146 w310] -> w118
          tunnel: [w145 w308] -> w116
          tunnel: [w144 w307] -> w115
          tunnel: [w143 w304] -> w114
          tunnel: [w141 w309] -> w113
          tunnel: [w140 w302] -> w112
          tunnel: [w138 TRUE] -> w111
          frame False {
            n43 = case shown="False" w158 {
              tunnel: w175 -> [_ w279]
              tunnel: [w221 w278] -> w154
              tunnel: w174 -> [w247 w277]
              tunnel: w173 -> [w245 w276]
              tunnel: [w240 w254] -> w137
              tunnel: [w222 w253] -> w171
              tunnel: [w230 w252] -> w170
              tunnel: [w220 w249] -> w148
              frame False {
                n44 = call-dynamic "Read Holding Registers.vi"("error in (no error)"=w245, "number of holding registers"=u16 7, "starting address"=u16 10, "Modbus master in"=w247) -> ("error out"=w194:errorcluster, "register values"=w242:u16[], "Modbus master out"=w195:refnum<class "Modbus Master.lvclass">)  [unwired: 5 in]
                n45 = call-dynamic "Read Holding Registers.vi"("error in (no error)"=w194, "number of holding registers"=u16 1, "starting address"=u16 28, "Modbus master in"=w195) -> ("error out"=w192:errorcluster, "register values"=w191:u16[], "Modbus master out"=w193:refnum<class "Modbus Master.lvclass">)  [unwired: 5 in]
                n46 = call-dynamic "Read Holding Registers.vi"("error in (no error)"=w192, "number of holding registers"=u16 1, "starting address"=u16 40, "Modbus master in"=w193) -> ("error out"=w227:errorcluster, "register values"=w224:u16[], "Modbus master out"=w228:refnum<class "Modbus Master.lvclass">)  [unwired: 5 in]
                n47 = Index Array(array=w191) -> (element=w190:u16)  [unwired: 1 in]
                n48 = Index Array(array=w224) -> (element=w198:u16)  [unwired: 1 in]
                n49 = call-dynamic "Read Holding Registers.vi"("error in (no error)"=w227, "number of holding registers"=u16 1, "starting address"=u16 310, "Modbus master in"=w228) -> ("error out"=w212:errorcluster, "register values"=w233:u16[], "Modbus master out"=w213:refnum<class "Modbus Master.lvclass">)  [unwired: 5 in]
                n50 = Index Array(array=w242) -> (element #1=w241:u16, element #2=w239:u16, element #3=w238:u16, element #4=w237:u16, element #5=w236:u16, element #6=w229:u16, element #7=w189:u16)  [unwired: 7 in]
                n51 = Index Array(array=w233) -> (element=w232:u16)  [unwired: 1 in]
                n52 = To Word Integer(number=w189) -> (16bit integer=w188:i16)
                n53 = call-dynamic "Read Holding Registers.vi"("error in (no error)"=w212, "number of holding registers"=u16 7, "starting address"=u16 320, "Modbus master in"=w213) -> ("error out"=w203:errorcluster, "register values"=w211:u16[], "Modbus master out"=w204:refnum<class "Modbus Master.lvclass">)  [unwired: 5 in]
                n54 = Index Array(array=w211) -> (element #1=w210:u16, element #2=w209:u16, element #3=w208:u16, element #7=w207:u16)  [unwired: 7 in, 3 out]
                n55 = Bundle By Name(cluster=T7 {"M000"=0.0, "M001"=0.0, "M002"=0.0, "M003"=0.0, "M004"=0.0, "M005"=0.0, "M006"=0.0, "M007"=0.0, "M008"=0.0, "M009"=0.0, "M010"=0.0, "M011"=0.0, "M012"=0.0, "M013"=0.0, "M014"=0.0, "M015"=0.0, "M016"=0.0, "M017"=0.0, "M018"=0.0, "M019"=0.0, "M020"=0.0, "M021"=0.0, "M022"=0.0, "M023"=0.0, "M024"=0.0, "M025"=0.0, "M026"=0.0, "M027"=0.0, "M028"=0.0, "M029"=0.0, "M030"=0.0, "M031"=0.0} ("Parametri di misura"), "M000"=w241, "M001"=w239, "M002"=w238, "M003"=w237, "M004"=w236, "M005"=w229, "M006"=w188, "M018"=w190, "M030"=w198) -> (w240:T7)
                n56 = Bundle By Name(cluster=T6 {"C000"=0.0, "C001"=0.0, "C002"=0.0, "C010"=0.0, "C011"=0.0, "C012"=0.0, "C014"=0.0, "C015"=0.0, "C016"=0.0, "C017"=0.0, "C018"=0.0, "C030"=0.0, "C050"=0.0, "C051"=0.0, "C052"=0.0, "C060"=0.0, "C061"=0.0, "C062"=0.0, "C063"=0.0, "C070"=0.0, "C072"=0.0, "C074"=0.0, "C090"=0.0, "C091"=0.0, "C092"=0.0, "C093"=0.0, "C094"=0.0, "C100"=0.0, "C101"=0.0, "C102"=0.0, "C103"=0.0, "C105"=0.0, "C106"=0.0, "C107"=0.0, "C108"=0.0, "C110"=0.0, "C111"=0.0, "C112"=0.0, "C120"=0.0, "C121"=0.0, "C122"=0.0, "C130"=0.0, "C131"=0.0, "C132"=0.0, "C133"=0.0, "C134"=0.0, "C135"=0.0, "C141"=0.0, "C142"=0.0, "C143"=0.0, "C150"=0.0, "C151"=0.0, "C153"=0.0, "C154"=0.0, "C155"=0.0, "C156"=0.0, "C157"=0.0, "C158"=0.0, "C159"=0.0, "C160"=0.0, "C161"=0.0, "C162"=0.0, "C163"=0.0, "C164"=0.0, "C165"=0.0, "C170"=0.0} ("Parametri di configurazione"), "C000"=w232, "C010"=w210, "C011"=w209, "C012"=w208, "C016"=w207) -> (w230:T6)
                n57 = call-dynamic "Read Holding Registers.vi"("error in (no error)"=w203, "number of holding registers"=u16 2, "starting address"=u16 60, "Modbus master in"=w204) -> ("error out"=w202:errorcluster, "register values"=w200:u16[], "Modbus master out"=w201:refnum<class "Modbus Master.lvclass">)  [unwired: 5 in]
                n58 = call-dynamic "Read Holding Registers.vi"("error in (no error)"=w202, "number of holding registers"=u16 1, "starting address"=u16 75, "Modbus master in"=w201) -> ("error out"=w220:errorcluster, "register values"=w217:u16[], "Modbus master out"=w221:refnum<class "Modbus Master.lvclass">)  [unwired: 5 in]
                n59 = Index Array(array=w200) -> (element #1=w199:u16, element #2=w187:u16)  [unwired: 2 in]
                n60 = Index Array(array=w217) -> (element=w216:u16)  [unwired: 1 in]
                n61 = Bundle By Name(cluster=T5 {"P000"=0.0, "P001"=0.0, "P002"=0.0, "P003"=0.0, "P004"=0.0, "P005"=0.0, "P006"=0.0, "P010"=0.0, "P011"=0.0, "P012"=0.0, "P013"=0.0, "P014"=0.0, "P015"=0.0, "P016"=0.0, "P030"=0.0, "P031"=0.0, "P032"=0.0, "P033"=0.0, "P034"=0.0, "P035"=0.0, "P036"=0.0, "P037"=0.0, "P038"=0.0, "P039"=0.0, "P040"=0.0, "P050"=0.0, "P051"=0.0, "P052"=0.0, "P053"=0.0, "P054"=0.0, "P055"=0.0, "P056"=0.0, "P057"=0.0, "P058"=0.0, "P059"=0.0, "P060"=0.0, "P061"=0.0, "P062"=0.0, "P070"=0.0, "P071"=0.0, "P073"=0.0, "P074"=0.0, "P076"=0.0, "P077"=0.0, "P079"=0.0, "P080"=0.0, "P082"=0.0, "P083"=0.0, "P084"=0.0, "P085"=0.0, "P086"=0.0, "P087"=0.0, "P088"=0.0, "P100"=0.0, "P101"=0.0, "P102"=0.0, "P103"=0.0, "P104"=0.0, "P110"=0.0, "P111"=0.0, "P120"=0.0, "P121"=0.0, "P122"=0.0, "P123"=0.0, "P124"=0.0, "P125"=0.0, "P126"=0.0, "P127"=0.0, "P128"=0.0, "P129"=0.0, "P130"=0.0, "P131"=0.0, "P132"=0.0, "P133"=0.0, "P134"=0.0, "P150"=0.0, "P151"=0.0, "P152"=0.0, "P153"=0.0, "P154"=0.0, "P155"=0.0, "P156"=0.0, "P157"=0.0, "P158"=0.0, "P170"=0.0, "P171"=0.0, "P172"=0.0, "P173"=0.0, "P174"=0.0, "P175"=0.0, "P176"=0.0, "P177"=0.0, "P178"=0.0, "P179"=0.0, "P180"=0.0, "P181"=0.0, "P182"=0.0, "P183"=0.0, "P184"=0.0, "P185"=0.0, "P186"=0.0, "P187"=0.0, "P188"=0.0, "P189"=0.0, "P190"=0.0, "P191"=0.0, "P192"=0.0, "P193"=0.0, "P194"=0.0, "P195"=0.0, "P196"=0.0, "P197"=0.0, "P198"=0.0, "P199"=0.0, "P211"=0.0, "P212"=0.0, "P213"=0.0, "P214"=0.0, "P215"=0.0, "P216"=0.0, "P217"=0.0, "P221"=0.0, "P222"=0.0, "P223"=0.0, "P224"=0.0, "P230"=0.0, "P231"=0.0, "P240"=0.0, "P250"=0.0, "P251"=0.0} ("Parametri di programmazione"), "P010"=w199, "P030"=w216, "P011"=w187) -> (w222:T5)
              }
              frame True {
                n62 = for {
                  tunnel: w279 -> [w294] mode=indexing
                  shift-right: [w291] -> w278
                  shift-left: w277 -> [w292]
                  shift-right: [w293] -> w249
                  shift-left: w276 -> [w295]
                  shift-right: [w288] -> w255
                  shift-left: i32[][] [] -> [w287]
                  n63 = Index Array(array=w294) -> (element #1=w290:i32, element #2=w286:i32)  [unwired: 2 in]
                  n64 = call-dynamic "Read Holding Registers.vi"("error in (no error)"=w295, "number of holding registers"=w286, "starting address"=w290, "Modbus master in"=w292) -> ("error out"=w293:errorcluster, "register values"=w281:u16[], "Modbus master out"=w291:refnum<class "Modbus Master.lvclass">)  [unwired: 5 in]
                  n65 = Initialize Array(0 ("element"), w286) -> (w282:i32[])
                  n66 = Equal?(x=w281, y=u16[] []) -> (x = y?=w283:bool)
                  n67 = Select(t=w282, s=w283, f=w281) -> (s? t:f=w280:i32[])
                  n68 = for {
                    tunnel: w280 -> [w297] mode=indexing
                    tunnel: w290 -> [w299]
                    tunnel: [w296] -> w289 mode=indexing
                    i -> [w300]
                    n69 = Add(x=w299, y=w300) -> (x+y=w298:i32)
                    n70 = Build Array(w298, w297) -> (w296:i32[])
                  }
                  n71 = Build Array (concatenate)(w287, w289) -> (w288:i32[][])
                }
                "N°reg_ValReg" <- w255
                n72 = Array Subset(array=w255, index (row)=0 ("index"), length (row)=32 ("length")) -> (w273:i32[][])  [unwired: 2 in]
                n73 = Array Subset(array=w255, index (row)=32 ("index"), length (row)=130 ("length")) -> (w264:i32[][])  [unwired: 2 in]
                n74 = Array Subset(array=w255, index (row)=162 ("index"), length (row)=66 ("length")) -> (w259:i32[][])  [unwired: 2 in]
                n75 = Select(t=0, s="mostra num registro", f=1 ("disabled index (col)")) -> (s? t:f=w269:i32)
                n76 = Select(t=0, s="mostra num registro", f=1 ("disabled index (col)")) -> (s? t:f=w268:i32)
                n77 = Select(t=0, s="mostra num registro", f=1 ("disabled index (col)")) -> (s? t:f=w256:i32)
                n78 = Index Array(array=w273, index (col)=w269) -> (element=w272:i32[])  [unwired: 1 in]
                n79 = Index Array(array=w264, index (col)=w268) -> (element=w265:i32[])  [unwired: 1 in]
                n80 = Index Array(array=w259, index (col)=w256) -> (element=w258:i32[])  [unwired: 1 in]
                n81 = Array To Cluster(array=w272) -> (cluster=w254:T9)
                n82 = Array To Cluster(array=w265) -> (cluster=w253:T10)
                n83 = Array To Cluster(array=w258) -> (cluster=w252:T11)
              }
            }
            "t" <- w148
            n84 = call-dynamic "Read Holding Registers.vi"("error in (no error)"=w148, "number of holding registers"=u16 1, "starting address"=u16 8, "Modbus master in"=w154) -> ("error out"=w139:errorcluster, "register values"=w151:u16[], "Modbus master out"=w149:refnum<class "Modbus Master.lvclass">)  [unwired: 5 in]
            n85 = Divide(x=w147, y=2400.0) -> (x/y=w168:dbl)
            n86 = Index Array(array=w151) -> (element=w150:u16)  [unwired: 1 in]
            n87 = local read "DCREG"() -> (w172:T2)
            n88 = Bundle By Name(cluster=w172, "Parametri di misura"=w137, "Parametri di programmazione"=w171, "Parametri di configurazione"=w170, "Codice allarme"=w150) -> (w140:T2)
            n89 = Unbundle By Name(w140) -> ("Parametri di misura.M004"=w136:dbl, "Parametri di misura.M006"=w135:dbl, "Parametri di misura.M018"=w134:dbl)
            "M004 I ARMATURA [A]" <- w136
            "M006 V ARMATURA [V]" <- w135
            n90 = Divide(x=w134, y=100.0) -> (x/y=→"M0018 I CAMPO [A]":dbl)
            n91 = Greater Or Equal?(x=w135, y=550.0) -> (x >= y?=w166:bool)
            n92 = Select(t=0.0, s=w166, f=w135) -> (s? t:f=w156:dbl)
            n93 = Multiply(x=w168, y=w136) -> (x*y=w161:dbl)
            n94 = Greater Or Equal?(x=w161, y=550.0) -> (x >= y?=w163:bool)
            n95 = Select(t=0.0, s=w163, f=w161) -> (s? t:f=w157:dbl)
            n96 = Equal To 0?(x=w156) -> (x = 0?=w155:bool)
            n97 = disable-structure shown="Enabled" {
              disable-tunnel: [w184 w186] -> w144
              disable-tunnel: [w180 w185] -> w145
              disable-tunnel: w157 -> [w179 w186]
              disable-tunnel: w156 -> [w178 w185]
              disable-tunnel: w155 -> [w177 _]
              frame Disabled {
                n98 = Equal To 0?(x=w179) -> (x = 0?=w183:bool)
                n99 = call <vilib>:"Mean PtByPt.vi"("x"=w179, "sample length"=2, "initialize"=w183) -> ("mean"=w184:dbl)  [unwired: 1 in, 1 out]
                n100 = call <vilib>:"Mean PtByPt.vi"("x"=w178, "sample length"=2, "initialize"=w177) -> ("mean"=w180:dbl)  [unwired: 1 in, 1 out]
              }
              frame Enabled {
              }
            }
            n101 = Multiply(x=w145, y=w144) -> (x*y=w160:dbl)
            n102 = Divide(x=w160, y=1000.0) -> (x/y=w143:dbl)
            n103 = Divide(x=w134, y=100.0) -> (x/y=w141:dbl)
            n104 = case shown="No Error" w139 {
              tunnel: [TRUE _] -> w138
              frame No Error {
              }
              frame Error {
              }
            }
          }
          frame True {
            n105 = local read "Imax mot"() -> (w307:dbl)
            n106 = local read "Vdcreg"() -> (w308:dbl)
            n107 = local read "Iecc"() -> (w309:dbl)
            n108 = Wait (ms)(milliseconds to wait=u32 200) -> ()  [unwired: 1 out]
            n109 = Multiply(x=w308, y=w307) -> (x*y=w306:dbl)
            n110 = Divide(x=w306, y=1000.0) -> (x/y=w304:dbl)
            n111 = local read "DCREG"() -> (w302:T2)
          }
        }
        "V[V]" <- w116
        "I[A]" <- w115
        "P[KW]" <- w114
        "Iecc" <- w113
        n112 = Bundle By Name(cluster=w112, "Comunicazione"=w111) -> (w107:T2)
        n113 = case shown="No Error" w117 {
          tunnel: [cluster{"String":string, "variant":variant} {"String"="READ", "variant"=variant} ("element") cluster{"String":string, "variant":variant} {"String"="INITIALIZE", "variant"=variant} ("element")] -> w119
          tunnel: [TRUE FALSE] -> w105
          frame No Error {
          }
          frame Error {
          }
        }
        n114 = local write "DCREG"(w107) -> ()
        n115 = Bundle By Name(cluster=T4 {"Array of elements"=[], "Single element"={"String"="READ DCREG", "variant"=variant}, "enque at\nopposite end (F)"=FALSE, "no replications (F)"=FALSE} ("Enqueue cluster"), "Single element.variant"=w107) -> (w110:T4)
        n116 = Enqueue Element(queue=w118, element=w119) -> ()  [unwired: 2 in, 3 out]
        n117 = local write "Connesso?"(w105) -> ()
        n118 = call <userlib>:"SMQ_MANAGER.vi"("Function"=enum16{"INITIALIZE", "ENQUEUE", "STOP ALL"}."ENQUEUE", "Queue name"="DATA_Q", "Enqueue cluster"=w110) -> ()  [unwired: 8 in, 1 out]
      }
      frame "IDLE" {
        n119 = case shown="False" w321 {
          tunnel: w323 -> [w327 _]
          tunnel: w322 -> [w326 _]
          frame False {
            n120 = call-dynamic "Close.vi"("error in (no error)"=w326, "Modbus master in"=w327) -> ("error out"=w325:errorcluster)  [unwired: 9 in]
            n121 = call <vilib>:"Clear Errors.vi"("error in (no error)"=w325) -> ()  [unwired: 5 in, 2 out]
          }
          frame True {
          }
        }
        n122 = Flush Queue(queue=w324) -> ()  [unwired: 1 in, 3 out]
        n123 = local read "DCREG"() -> (w316:T2)
        n124 = Bundle By Name(cluster=w316, "Comunicazione"=FALSE) -> (w315:T2)
        n125 = Bundle By Name(cluster=T4 {"Array of elements"=[], "Single element"={"String"="READ DCREG", "variant"=variant}, "enque at\nopposite end (F)"=FALSE, "no replications (F)"=FALSE} ("Enqueue cluster"), "Single element.variant"=w315) -> (w319:T4)
        n126 = call <userlib>:"SMQ_MANAGER.vi"("Function"=enum16{"INITIALIZE", "ENQUEUE", "STOP ALL"}."ENQUEUE", "Queue name"="DATA_Q", "Enqueue cluster"=w319) -> ()  [unwired: 8 in, 1 out]
        "Connesso?" <- FALSE
      }
      frame "WRITE REGISTER" {
        n127 = call-dynamic "Write Multiple Holding Registers.vi"("holding register values"="holding register values", "starting address"="starting address", "Modbus master in"=w334) -> ("Modbus master out"=w331:refnum<class "Modbus Master.lvclass">)  [unwired: 7 in, 1 out]
        n128 = Enqueue Element(queue=w328, element=cluster{"String":string, "variant":variant} {"String"="READ", "variant"=variant}, error in (no error)=w329) -> ()  [unwired: 1 in, 3 out]
      }
      frame "IngDig=0" {
        n129 = Build Array(u16 0 ("starting address")) -> (w339:u16[])
        n130 = call-dynamic "Write Multiple Holding Registers.vi"("error in (no error)"=w335, "holding register values"=w339, "starting address"=u16 40, "Modbus master in"=w336) -> ("error out"=w338:errorcluster, "Modbus master out"=w342:refnum<class "Modbus Master.lvclass">)  [unwired: 6 in]
        n131 = Enqueue Element(queue=w343, element=cluster{"String":string, "variant":variant} {"String"="READ", "variant"=variant}, error in (no error)=w338) -> (error out=w337:errorcluster)  [unwired: 1 in, 2 out]
      }
      frame "Rif_Vel" {
        n132 = local read "P011 Vdc arm NOM"() -> (w348:dbl)
        n133 = global read "Global FINE AVVIO.vi" "vARM NOM DC"() -> (w349:dbl)
        n134 = Variant To Data(error in=w368, type=0.0 ("starting address"), Variant=w366) -> (data=w347:dbl, error out=w367:errorcluster)
        "Vdcreg" <- w347
        n135 = Divide(x=w349, y=w348) -> (x/y=w345:dbl)
        n136 = Multiply(x=w347, y=w345) -> (x*y=w346:dbl)
        n137 = local read "P010 RPM max"() -> (w352:dbl)
        n138 = In Range and Coerce(upper limit=w352, x=w346, lower limit=0.0) -> (coerced(x)=w354:dbl)  [unwired: 1 out]
        n139 = Divide(x=w354, y=w352) -> (x/y=w357:dbl)
        n140 = Multiply(x=w357, y=100.0) -> (x*y=w362:dbl)
        n141 = Multiply(x=16383.0, y=w362) -> (x*y=w360:dbl)
        n142 = Divide(x=w360, y=100.0) -> (x/y=w356:dbl)
        n143 = Flush Queue(queue=w351) -> (queue out=w350:refnum<queue>)  [unwired: 1 in, 2 out]
        n144 = case shown="False" w355 {
          tunnel: [w376 w379] -> w370
          tunnel: w367 -> [w375 w379]
          tunnel: w364 -> [w374 w380]
          tunnel: [w373 w380] -> w363
          tunnel: w356 -> [w372 _]
          frame False {
            n145 = Build Array(w372) -> (w377:dbl[])
            n146 = call-dynamic "Write Multiple Holding Registers.vi"("error in (no error)"=w375, "holding register values"=w377, "starting address"=u16 25, "Modbus master in"=w374) -> ("error out"=w376:errorcluster, "Modbus master out"=w373:refnum<class "Modbus Master.lvclass">)  [unwired: 6 in]
          }
          frame True {
          }
        }
        n147 = Enqueue Element(queue=w350, element=cluster{"String":string, "variant":variant} {"String"="READ", "variant"=variant}, error in (no error)=w370) -> (error out=w369:errorcluster)  [unwired: 1 in, 2 out]
      }
      frame "Imax_mot" {
        n148 = Variant To Data(type=0.0 ("starting address"), Variant=w393) -> (data=w383:dbl, error out=w395:errorcluster)  [unwired: 1 in]
        "Imax mot" <- w383
        n149 = Flush Queue(queue=w387) -> (queue out=w386:refnum<queue>)  [unwired: 1 in, 2 out]
        n150 = Divide(x=w383, y=w382) -> (x/y=w384:dbl)
        n151 = Multiply(x=w384, y=100.0) -> (x*y=w381:dbl)
        n152 = Build Array(w381) -> (w396:dbl[])
        n153 = call-dynamic "Write Multiple Holding Registers.vi"("error in (no error)"=w395, "holding register values"=w396, "starting address"=u16 310, "Modbus master in"=w392) -> ("error out"=w389:errorcluster, "Modbus master out"=w391:refnum<class "Modbus Master.lvclass">)  [unwired: 6 in]
        n154 = Enqueue Element(queue=w386, element=cluster{"String":string, "variant":variant} {"String"="READ", "variant"=variant}, error in (no error)=w389) -> (error out=w388:errorcluster)  [unwired: 1 in, 2 out]
      }
      frame "Iecc" {
        n155 = Variant To Data(type=0.0 ("starting address"), Variant=w408) -> (data=w404:dbl, error out=w412:errorcluster)  [unwired: 1 in]
        "Iecc" <- w404
        n156 = Divide(x=w404, y=w403) -> (x/y=w402:dbl)
        n157 = Multiply(x=w402, y=1000.0) -> (x*y=w400:dbl)
        n158 = Flush Queue(queue=w399) -> (queue out=w398:refnum<queue>)  [unwired: 1 in, 2 out]
        n159 = case shown="False" w405 {
          tunnel: w412 -> [w418 w421]
          tunnel: [w417 w421] -> w409
          tunnel: w407 -> [w416 w422]
          tunnel: [w415 w422] -> w406
          tunnel: w400 -> [w414 _]
          frame False {
            n160 = Build Array(w414) -> (w419:dbl[])
            n161 = call-dynamic "Write Multiple Holding Registers.vi"("error in (no error)"=w418, "holding register values"=w419, "starting address"=u16 320, "Modbus master in"=w416) -> ("error out"=w417:errorcluster, "Modbus master out"=w415:refnum<class "Modbus Master.lvclass">)  [unwired: 6 in]
          }
          frame True {
          }
        }
        n162 = Enqueue Element(queue=w398, element=cluster{"String":string, "variant":variant} {"String"="READ", "variant"=variant}, error in (no error)=w409) -> ()  [unwired: 1 in, 3 out]
      }
      frame "Config DCREG" {
        w436 = 35.0  # I ecc nom azionamento
        w435 = 900.0  # Iarm nom azionamento
        # "attenzione! il dcreg non si configura se il teleruttore di potenza è chiuso"
        n163 = local read "Configurazioni dcreg"() -> (w424:T1)
        n164 = Unbundle By Name(w424) -> ("P010 RPM max"=w423:dbl, "P011 Vdc arm NOM"=w461:dbl, "C000 Iarm NOM"=w441:dbl, "C010 Iecc NOM"=w438:dbl)
        "P011 Vdc arm NOM" <- w461
        "P010 RPM max" <- w423
        n165 = In Range and Coerce(upper limit=6000.0, x=w423, lower limit=300.0) -> (coerced(x)=w464:dbl)  [unwired: 1 out]
        n166 = In Range and Coerce(upper limit=2000.0, x=w461, lower limit=50.0) -> (coerced(x)=w460:dbl)  [unwired: 1 out]
        n167 = To Unsigned Word Integer(number=w464) -> (unsigned 16bit integer=w459:u16)
        n168 = To Unsigned Word Integer(number=w460) -> (unsigned 16bit integer=w431:u16)
        n169 = In Range and Coerce(upper limit=w435, x=w441, lower limit=0.0) -> (coerced(x)=w440:dbl)  [unwired: 1 out]
        n170 = Build Array(w431) -> (w430:u16[])
        n171 = Build Array(w459) -> (w458:u16[])
        n172 = call-dynamic "Write Multiple Holding Registers.vi"("holding register values"=w458, "starting address"=u16 60, "Modbus master in"=w457) -> ("error out"=w425:errorcluster, "Modbus master out"=w433:refnum<class "Modbus Master.lvclass">)  [unwired: 7 in]
        "error out 5" <- w425
        n173 = call-dynamic "Write Multiple Holding Registers.vi"("holding register values"=w430, "starting address"=u16 61, "Modbus master in"=w433) -> ("error out"=w427:errorcluster, "Modbus master out"=w432:refnum<class "Modbus Master.lvclass">)  [unwired: 7 in]
        "error out 2" <- w427
        n174 = Divide(x=w440, y=w435) -> (x/y=w453:dbl)
        n175 = In Range and Coerce(upper limit=w436, x=w438, lower limit=0.0) -> (coerced(x)=w437:dbl)  [unwired: 1 out]
        n176 = Multiply(x=w453, y=100.0) -> (x*y=w452:dbl)
        n177 = To Unsigned Word Integer(number=w452) -> (unsigned 16bit integer=w451:u16)
        n178 = Build Array(w451) -> (w455:u16[])
        n179 = call-dynamic "Write Multiple Holding Registers.vi"("holding register values"=w455, "starting address"=u16 310, "Modbus master in"=w432) -> ("error out"=w428:errorcluster, "Modbus master out"=w446:refnum<class "Modbus Master.lvclass">)  [unwired: 7 in]
        "error out 3" <- w428
        n180 = Divide(x=w437, y=w436) -> (x/y=w450:dbl)
        n181 = Multiply(x=w450, y=1000.0) -> (x*y=w444:dbl)
        n182 = To Unsigned Word Integer(number=w444) -> (unsigned 16bit integer=w443:u16)
        n183 = Build Array(w443) -> (w447:u16[])
        n184 = call-dynamic "Write Multiple Holding Registers.vi"("holding register values"=w447, "starting address"=u16 320, "Modbus master in"=w446) -> ("error out"=w429:errorcluster, "Modbus master out"=w445:refnum<class "Modbus Master.lvclass">)  [unwired: 7 in]
        "error out 4" <- w429
        n185 = Merge Errors(w429, w428, w427, w425) -> (w426:errorcluster)
      }
      frame "Configurazioni DCREG" {
        n186 = Variant To Data(type=T1 {"P011 Vdc arm NOM"=0.0, "C000 Iarm NOM"=0.0, "C010 Iecc NOM"=0.0, "P010 RPM max"=0.0} ("Config DCreg"), Variant=w471) -> (data=→"Configurazioni dcreg":T1)  [unwired: 1 in, 1 out]
        n187 = local read "Connesso?"() -> (w469:bool)
        n188 = case shown="True" w469 {
          tunnel: w468 -> [_ w475]
          frame False {
          }
          frame True {
            n189 = Enqueue Element(queue=w475, element=cluster{"String":string, "variant":variant} {"String"="Config DCREG", "variant"=variant}) -> ()  [unwired: 2 in, 3 out]
          }
        }
      }
      frame "Imposta deflussaggio" {
        n190 = Variant To Data(type=T8 {"C011"=0.0, "C012"=0.0, "C016"=0.0, "Conferma"=FALSE} ("Value"), Variant=w495) -> (data=w493:T8)  [unwired: 1 in, 1 out]
        n191 = Unbundle By Name(w493) -> ("C011"=w489:dbl, "C012"=w488:dbl, "C016"=w484:dbl)
        n192 = To Unsigned Word Integer(number=w489) -> (unsigned 16bit integer=w487:u16)
        n193 = To Unsigned Word Integer(number=w488) -> (unsigned 16bit integer=w486:u16)
        n194 = To Unsigned Word Integer(number=w484) -> (unsigned 16bit integer=w483:u16)
        n195 = Build Array(w487, w486) -> (w485:u16[])
        n196 = Build Array(w483) -> (w477:u16[])
        n197 = call-dynamic "Write Multiple Holding Registers.vi"("error in (no error)"=w490, "holding register values"=w485, "starting address"=u16 321, "Modbus master in"=w491) -> ("error out"=w479:errorcluster, "Modbus master out"=w481:refnum<class "Modbus Master.lvclass">)  [unwired: 6 in]
        n198 = call-dynamic "Write Multiple Holding Registers.vi"("error in (no error)"=w479, "holding register values"=w477, "starting address"=u16 326, "Modbus master in"=w481) -> ("error out"=w478:errorcluster, "Modbus master out"=w480:refnum<class "Modbus Master.lvclass">)  [unwired: 6 in]
      }
      frame "IngDig=1" {
        n199 = Build Array(u16 1 ("starting address")) -> (w502:u16[])
        n200 = call-dynamic "Write Multiple Holding Registers.vi"("error in (no error)"=w500, "holding register values"=w502, "starting address"=u16 40, "Modbus master in"=w501) -> ("error out"=w497:errorcluster, "Modbus master out"=w499:refnum<class "Modbus Master.lvclass">)  [unwired: 6 in]
        n201 = Enqueue Element(queue=w498, element=cluster{"String":string, "variant":variant} {"String"="READ", "variant"=variant}, error in (no error)=w497) -> (error out=w496:errorcluster)  [unwired: 1 in, 2 out]
      }
      frame "IngDig=2" {
        n202 = Build Array(u16 2 ("starting address")) -> (w512:u16[])
        n203 = call-dynamic "Write Multiple Holding Registers.vi"("error in (no error)"=w511, "holding register values"=w512, "starting address"=u16 40, "Modbus master in"=w510) -> ("error out"=w507:errorcluster, "Modbus master out"=w509:refnum<class "Modbus Master.lvclass">)  [unwired: 6 in]
        n204 = Enqueue Element(queue=w508, element=cluster{"String":string, "variant":variant} {"String"="READ", "variant"=variant}, error in (no error)=w507) -> (error out=w506:errorcluster)  [unwired: 1 in, 2 out]
      }
      frame "IngDig=3" {
        w524 = u16 40 ("starting address")
        n205 = Build Array(u16 3 ("starting address")) -> (w533:u16[])
        n206 = call-dynamic "Write Multiple Holding Registers.vi"("error in (no error)"=w532, "holding register values"=w533, "starting address"=w524, "Modbus master in"=w531) -> ("error out"=w528:errorcluster, "Modbus master out"=w526:refnum<class "Modbus Master.lvclass">)  [unwired: 6 in]
        n207 = call-dynamic "Read Holding Registers.vi"("error in (no error)"=w528, "number of holding registers"=u16 1, "starting address"=w524, "Modbus master in"=w526) -> ("error out"=w527:errorcluster, "register values"=w522:u16[], "Modbus master out"=w525:refnum<class "Modbus Master.lvclass">)  [unwired: 5 in]
        n208 = Index Array(array=w522) -> (element=w521:u16)  [unwired: 1 in]
        n209 = Equal?(x=w521, y=u16 3) -> (x = y?=w519:bool)
        n210 = Select(t=cluster{"String":string, "variant":variant} {"String"="READ", "variant"=variant} ("element"), s=w519, f=cluster{"String":string, "variant":variant} {"String"="IngDig=3", "variant"=variant} ("element")) -> (s? t:f=w517:cluster{"String":string, "variant":variant})
        n211 = Enqueue Element(queue=w530, element=w517, error in (no error)=w527) -> (error out=w529:errorcluster)  [unwired: 1 in, 2 out]
      }
      frame "fino a 20kw" {
        n212 = case shown="True" FALSE {
          tunnel: w542 -> [w545 w558]
          tunnel: [w543 w557] -> w541
          tunnel: [w544 w559] -> w540
          tunnel: w539 -> [w544 w547]
          tunnel: w538 -> [w543 w546]
          tunnel: [w545 w558] -> w536
          frame False {
          }
          frame True {
            # "KpCurr\nTintDisc\nTintCont"
            n213 = flat-sequence {
              tunnel: w546 -> [w564]
              tunnel: w547 -> [w562]
              tunnel: [w563] -> w556
              tunnel: [w561] -> w555
              tunnel: [w568] -> w551
              tunnel: [w569] -> w552
              tunnel: w556 -> [w569]
              tunnel: w555 -> [w568]
              frame #0 {
                # "anello corrente"
                n214 = Build Array(u16 1 ("Register")) -> (w566:u16[])
                n215 = call-dynamic "Write Multiple Holding Registers.vi"("error in (no error)"=w564, "holding register values"=w566, "starting address"=u16 336, "Modbus master in"=w562) -> ("error out"=w563:errorcluster, "Modbus master out"=w561:refnum<class "Modbus Master.lvclass">)  [unwired: 6 in]
              }
              frame #1 {
                n216 = Wait (ms)(milliseconds to wait=u16 200 ("starting address")) -> ()  [unwired: 1 out]
              }
            }
            n217 = Build Array(u16 400 ("starting address"), u16 5000 ("starting address"), u16 10000 ("starting address")) -> (w553:u16[])
            n218 = call-dynamic "Write Multiple Holding Registers.vi"("error in (no error)"=w552, "holding register values"=w553, "starting address"=u16 135, "Modbus master in"=w551) -> ("error out"=w557:errorcluster, "Modbus master out"=w559:refnum<class "Modbus Master.lvclass">)  [unwired: 6 in]
          }
        }
        n219 = Enqueue Element(queue=w536, element=cluster{"String":string, "variant":variant} {"String"="READ", "variant"=variant}) -> ()  [unwired: 2 in, 3 out]
      }
      frame "superiore a 20kw" {
        n220 = case shown="True" FALSE {
          tunnel: [w579 w592] -> w576
          tunnel: [w578 w591] -> w575
          tunnel: w572 -> [w578 w581]
          tunnel: w571 -> [w579 w580]
          frame False {
          }
          frame True {
            n221 = flat-sequence {
              tunnel: w581 -> [w596]
              tunnel: w580 -> [w595]
              tunnel: [w598] -> w590
              tunnel: [w597] -> w589
              tunnel: [w601] -> w584
              tunnel: [w602] -> w586
              tunnel: w590 -> [w602]
              tunnel: w589 -> [w601]
              frame #0 {
                # "anello corrente"
                n222 = Build Array(u16 0 ("Register")) -> (w593:u16[])
                n223 = call-dynamic "Write Multiple Holding Registers.vi"("error in (no error)"=w595, "holding register values"=w593, "starting address"=u16 336, "Modbus master in"=w596) -> ("error out"=w598:errorcluster, "Modbus master out"=w597:refnum<class "Modbus Master.lvclass">)  [unwired: 6 in]
              }
              frame #1 {
                n224 = Wait (ms)(milliseconds to wait=u32 200) -> ()  [unwired: 1 out]
              }
            }
            n225 = Build Array(u16 4000 ("starting address"), u16 130 ("starting address"), u16 3200 ("starting address")) -> (w587:u16[])
            n226 = call-dynamic "Write Multiple Holding Registers.vi"("error in (no error)"=w586, "holding register values"=w587, "starting address"=u16 135, "Modbus master in"=w584) -> ("error out"=w592:errorcluster, "Modbus master out"=w591:refnum<class "Modbus Master.lvclass">)  [unwired: 6 in]
          }
        }
        n227 = Enqueue Element(queue=w573, element=cluster{"String":string, "variant":variant} {"String"="READ", "variant"=variant}, error in (no error)=w576) -> (error out=w574:errorcluster)  [unwired: 1 in, 2 out]
      }
      frame "Imposta rampa" {
        n228 = Variant To Data(type=0.0, Variant=w622) -> (data=w608:dbl)  [unwired: 1 in, 1 out]
        n229 = Multiply(x=w608, y=100.0) -> (x*y=w606:dbl)
        n230 = Build Array(w606, w606, w606, w606) -> (w620:dbl[])
        n231 = Equal To 0?(x=w608) -> (x = 0?=w611:bool)
        n232 = call-dynamic "Write Multiple Holding Registers.vi"("error in (no error)"=w617, "holding register values"=w620, "starting address"=u16 75, "Modbus master in"=w619) -> ("error out"=w615:errorcluster, "Modbus master out"=w613:refnum<class "Modbus Master.lvclass">)  [unwired: 6 in]
        n233 = Select(t=0.1, s=w611, f=w608) -> (s? t:f=w605:dbl)
        n234 = Multiply(x=10.0, y=w605) -> (x*y=w603:dbl)
        n235 = Build Array(w603) -> (w610:dbl[])
        n236 = call-dynamic "Write Multiple Holding Registers.vi"("error in (no error)"=w615, "holding register values"=w610, "starting address"=u16 85, "Modbus master in"=w613) -> ("error out"=w614:errorcluster, "Modbus master out"=w612:refnum<class "Modbus Master.lvclass">)  [unwired: 6 in]
      }
      frame "Exit" {
        n237 = property on="stop" class="Bool"("Val(Sgnl)"=TRUE) -> ()  [unwired: 2 in, 2 out]
      }
    }
    "Numeric" <- w64
  }
  n238 = while {
    tunnel: w41 -> [w628]
    stop <- w627 stop-if-true
    # "PROCESSI A EVENTI"
    n239 = event shown="[5] \"set Iarm\": Value Change" {
      selector: _ -> [_ _ _ _ _ _ _ _ _]
      dyn-events: _ -> [_ _ _ _ _ _ _ _ _]
      timeout: _ -> [_ _ _ _ _ _ _ _ _]
      tunnel: w628 -> [w630 w632 w635 w637 w642 w646 w650 w654 w656]
      tunnel: [_ TRUE _ _ _ _ _ _ _] -> w627
      event "write register": Value Change {
        n240 = event-data() -> ()  [unwired: 1 in, 2 out]
        n241 = Flush Queue(queue=w630) -> (error out=w629:errorcluster)  [unwired: 1 in, 2 out]
        n242 = Enqueue Element(queue=w630, element=cluster{"String":string, "variant":variant} {"String"="WRITE REGISTER", "variant"=variant}, error in (no error)=w629) -> ()  [unwired: 1 in, 3 out]
      }
      event "stop": Value Change {
        n243 = event-data() -> ()  [unwired: 1 in, 2 out]
        n244 = Enqueue Element(queue=w632, element=cluster{"String":string, "variant":variant} {"String"="Exit", "variant"=variant}) -> ()  [unwired: 2 in, 3 out]
      }
      event "connetti": Value Change {
        n245 = event-data() -> ()  [unwired: 1 in, 2 out]
        n246 = Enqueue Element(queue=w635, element=cluster{"String":string, "variant":variant} {"String"="INITIALIZE", "variant"=variant}) -> ()  [unwired: 2 in, 3 out]
      }
      event "disconnetti": Value Change {
        n247 = event-data() -> ()  [unwired: 1 in, 2 out]
        n248 = Enqueue Element(queue=w637, element=cluster{"String":string, "variant":variant} {"String"="IDLE", "variant"=variant}) -> ()  [unwired: 2 in, 3 out]
      }
      event "set varm": Value Change {
        n249 = event-data() -> ()  [unwired: 1 in, 2 out]
        n250 = Bundle By Name(cluster=cluster{"String":string, "variant":variant} {"String"="Rif_Vel", "variant"=variant} ("element"), "variant"="Vdc arm") -> (w639:cluster{"String":string, "variant":variant})
        n251 = Enqueue Element(queue=w642, element=w639) -> ()  [unwired: 2 in, 3 out]
      }
      event "set Iarm": Value Change {
        n252 = event-data() -> ()  [unwired: 1 in, 2 out]
        n253 = Bundle By Name(cluster=cluster{"String":string, "variant":variant} {"String"="Imax_mot", "variant"=variant} ("element"), "variant"="Inom arm") -> (w644:cluster{"String":string, "variant":variant})
        n254 = Enqueue Element(queue=w646, element=w644) -> ()  [unwired: 2 in, 3 out]
      }
      event "set rampa": Value Change {
        n255 = event-data() -> ()  [unwired: 1 in, 2 out]
        n256 = Bundle By Name(cluster=cluster{"String":string, "variant":variant} {"String"="Imposta rampa", "variant"=variant} ("element"), "variant"="Rampa s") -> (w648:cluster{"String":string, "variant":variant})
        n257 = Enqueue Element(queue=w650, element=w648) -> ()  [unwired: 2 in, 3 out]
      }
      event "SET IECC": Value Change {
        n258 = event-data() -> ()  [unwired: 1 in, 2 out]
        n259 = Bundle By Name(cluster=cluster{"String":string, "variant":variant} {"String"="Iecc", "variant"=variant} ("element"), "variant"="IECC") -> (w652:cluster{"String":string, "variant":variant})
        n260 = Enqueue Element(queue=w654, element=w652) -> ()  [unwired: 2 in, 3 out]
      }
      event "config": Value Change {
        n261 = event-data() -> ()  [unwired: 1 in, 2 out]
        n262 = Bundle By Name(cluster=cluster{"String":string, "variant":variant} {"String"="Config DCREG", "variant"=variant} ("element"), "variant"="Config DCreg") -> (w657:cluster{"String":string, "variant":variant})
        n263 = Enqueue Element(queue=w656, element=w657) -> ()  [unwired: 2 in, 3 out]
      }
    }
  }
  n264 = call-dynamic "Close.vi"("error in (no error)"=w37, "Modbus master in"=w38) -> ("error out"=w36:errorcluster)  [unwired: 9 in]
  n265 = call <vilib>:"Clear Errors.vi"("error in (no error)"=w36) -> ("error out"=→"error out":errorcluster)  [unwired: 5 in, 1 out]
